vi "Initialize.vi"(7 "큐 입력":refnum<queue>, 8 "error in":errorcluster caption="에러 입력(에러 없음)", 11 "입력 클러스터":T1) -> (0 "error out":errorcluster caption="에러 출력", 2 "data 2 (3d)":string[][][](array[string]), 3 "data 1 (2d)":string[][](array[string]), 4 "Load?":bool)   [LabVIEW 2020]
uses:
  Controls/Clst_Initialize Input.ctl
  Controls/Cmd_Var Data IO.ctl
  Controls/Cmd_File path.ctl
  Controls/Cmd_File Type.ctl
  Variables/Global_Cal Info.vi
  Public/Polymorph/Table Initialize_2D.vi
  Public/Polymorph/Cell Space_Table.vi
  Public/Polymorph/String content_Str.vi
  Public/Polymorph/String content_Combo.vi
  Public/Polymorph/Table Initialize_Str.vi
  Public/Polymorph/Array Dedup_1D Str.vi
  Variables/Global_Cal STD.vi
  Public/Polymorph/Data Class_2D Str.vi
  <vilib>/Utility/file.llb/Read Delimited Spreadsheet (string).vi
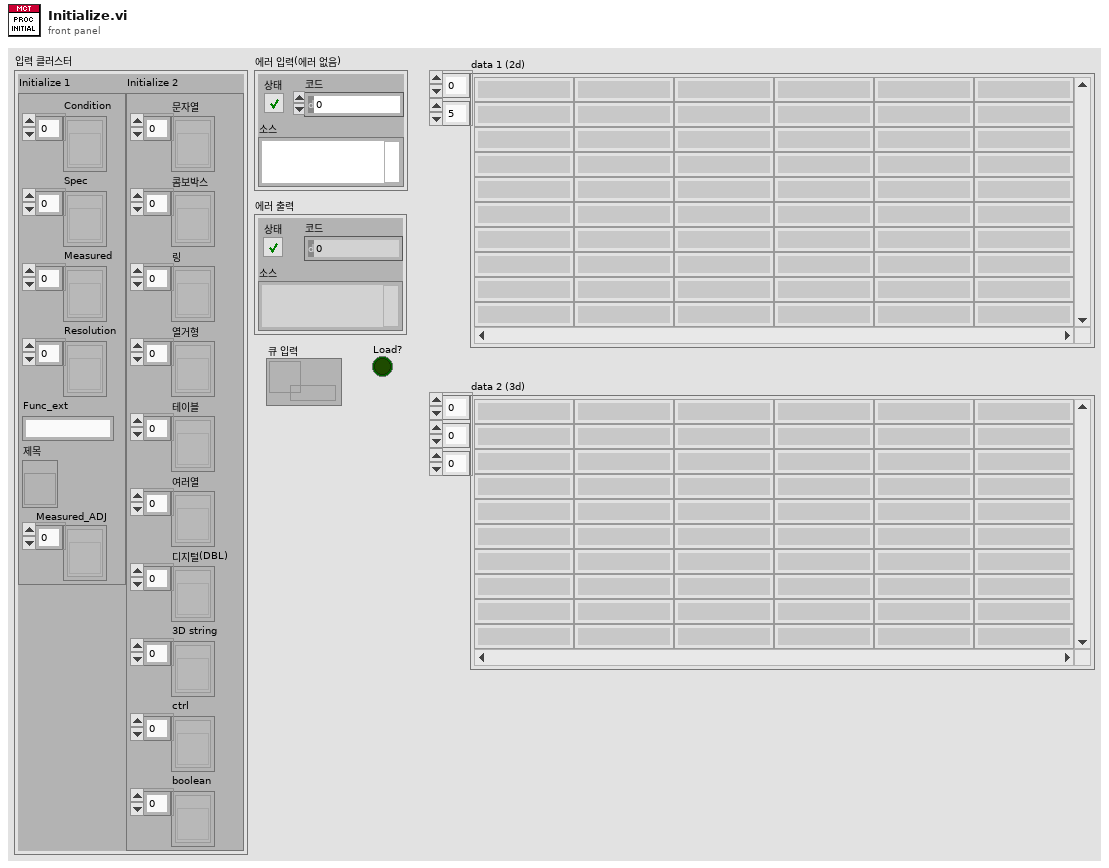
[diagram p1: front panel]
types:
  T1 = typedef "Clst_Initialize Input.ctl" = cluster{"Initialize 1":cluster{"Condition":refnum<vi>[], "Spec":refnum<vi>[], "Measured":refnum<vi>[], "Resolution":refnum<vi>[], "Func_ext":string, "제목":refnum<vi>, "Measured_ADJ":refnum<vi>[]}, "Initialize 2":cluster{"문자열":refnum<vi>[], "콤보박스":refnum<vi>[], "링":refnum<vi>[], "열거형":refnum<vi>[], "테이블":refnum<vi>[], "여러열":refnum<vi>[], "디지털(DBL)":refnum<vi>[], "3D string":refnum<vi>[], "ctrl":refnum<vi>[], "boolean":refnum<vi>[]}}
  T2 = cluster{"세부분류코드":string, "형식":string, "옵션":string, "측정기명":string, "EXCEL파일명":string, "TEMP":string}
  T3 = cluster{"Display sys":string[], "변경항목비활성":i32[], "추가항목비활성":i32[]}
  T4 = typedef "Cmd_Var Data IO.ctl" = enum16{"Condition", "Condition Default", "Condition_Temp", "Resolution", "Resolution Default", "Resolution Old", "Spec", "Spec Default", "Spec Old", "Spec Temp", "Result", "Result2", "Result3", "Result_Temp", "Result_ADJ", "Result_ADJ2", "STD1", "STD2", "STD3", "STD4", "STD5", "STD Temp", "CMC", "CMC Default"}
  T5 = enum8{"Enabled", "Disabled", "Disabled and Grayed Out"}
  T6 = typedef "Cmd_File Type.ctl" = enum16{"엑셀", "엑셀(2003)", "텍스트", "설정", "2진", "VI", "CSV", "LOG", "폴더"}
  T7 = typedef "Clst_Get Calproc.ctl" = cluster{"제목":string, "Condition":string[][], "Resolution":string[][], "Spec":string[][], "Data":string[][], "CMC":string[][], "NumRows":u32, "Temp_1":string[][]}
  T8 = typedef "Cmd_File path.ctl" = enum16{"에러로그", "데이터파일경로", "성적서원본", "지난성적서", "Data Files", "경로생성", "Updater", "Template", "설정파일경로", "FTP Upload", "Update 경로", "어플리케이션"}
  T9 = typedef "Clst_Cal Info Global.ctl" = cluster{"등록번호":string, "의뢰기관":string, "기기명":string, "제작회사":string, "형식":string, "기기번호":string, "소분류코드":string, "세부분류코드":string, "교정주기":string, "접수번호":string, "교정일자":string, "교정절차서 1":string, "교정절차서 2":string, "교정절차서 3":string, "접수확인자":string, "인증교정자":string, "기술책임자":string, "KOLAS 유무":string, "진행상태":string, "의뢰기관코드":string, "입고형태":string, "영문성적서?":bool, "합불판정?":bool, "부록?":bool, "절차서번호 1":string, "절차서번호 2":string, "절차서번호 3":string, "교정방식":string, "부서명":string}
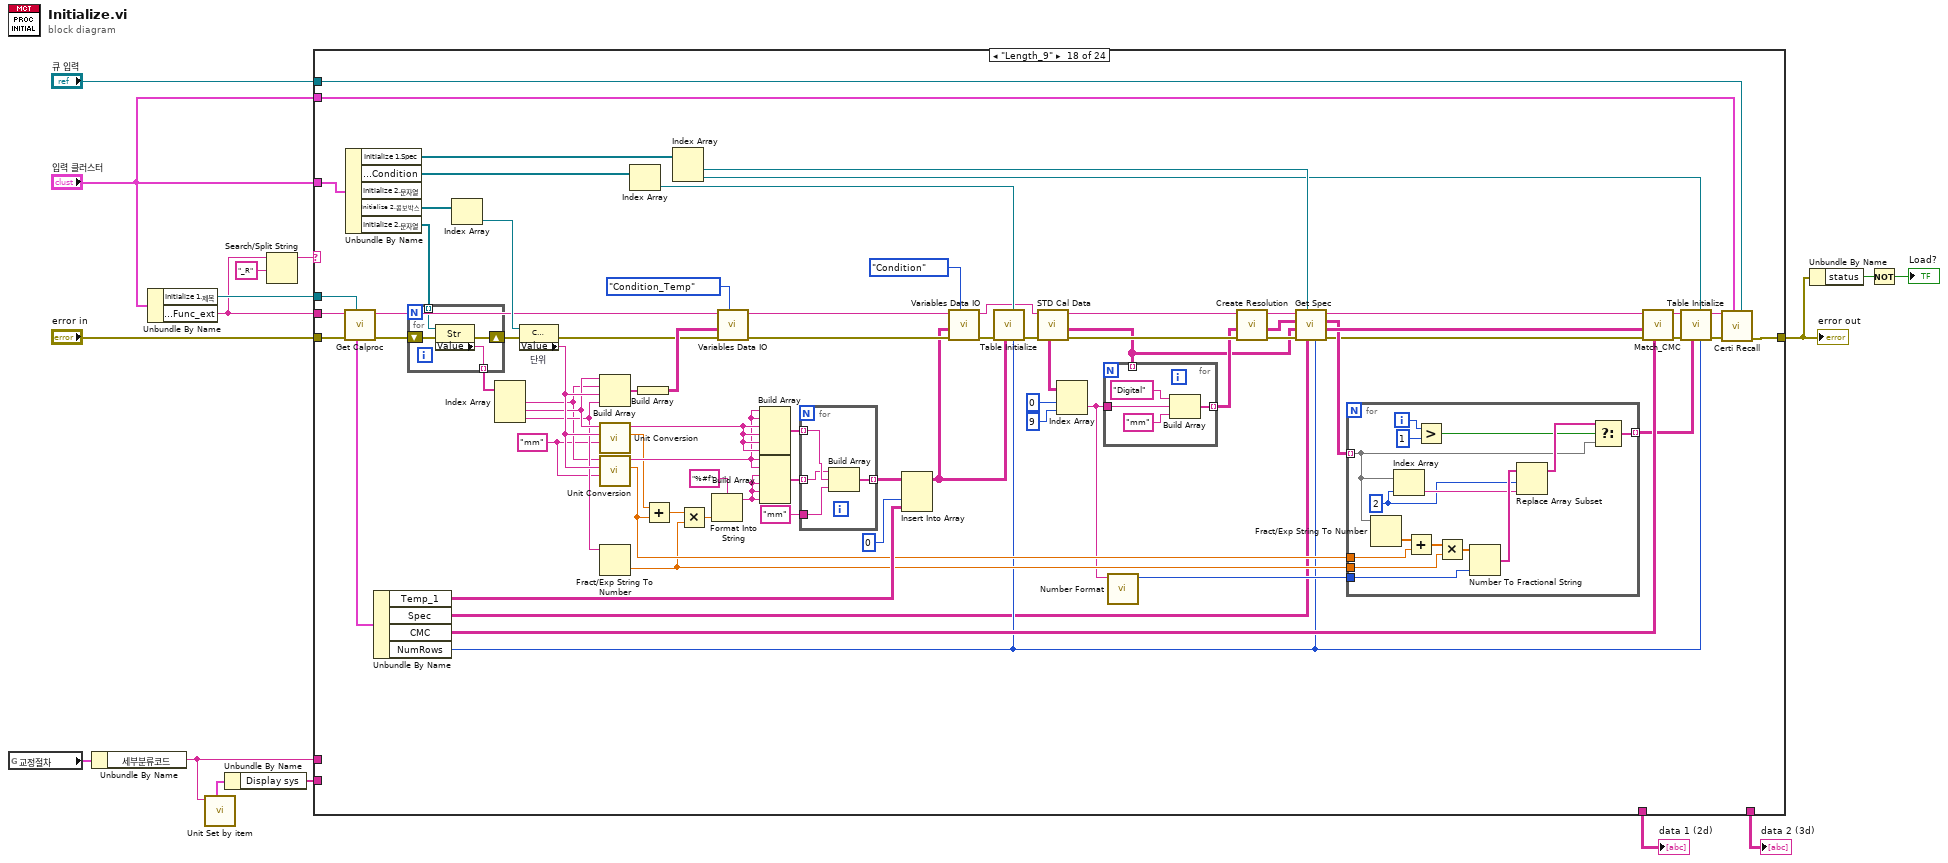
[diagram p0: block diagram]
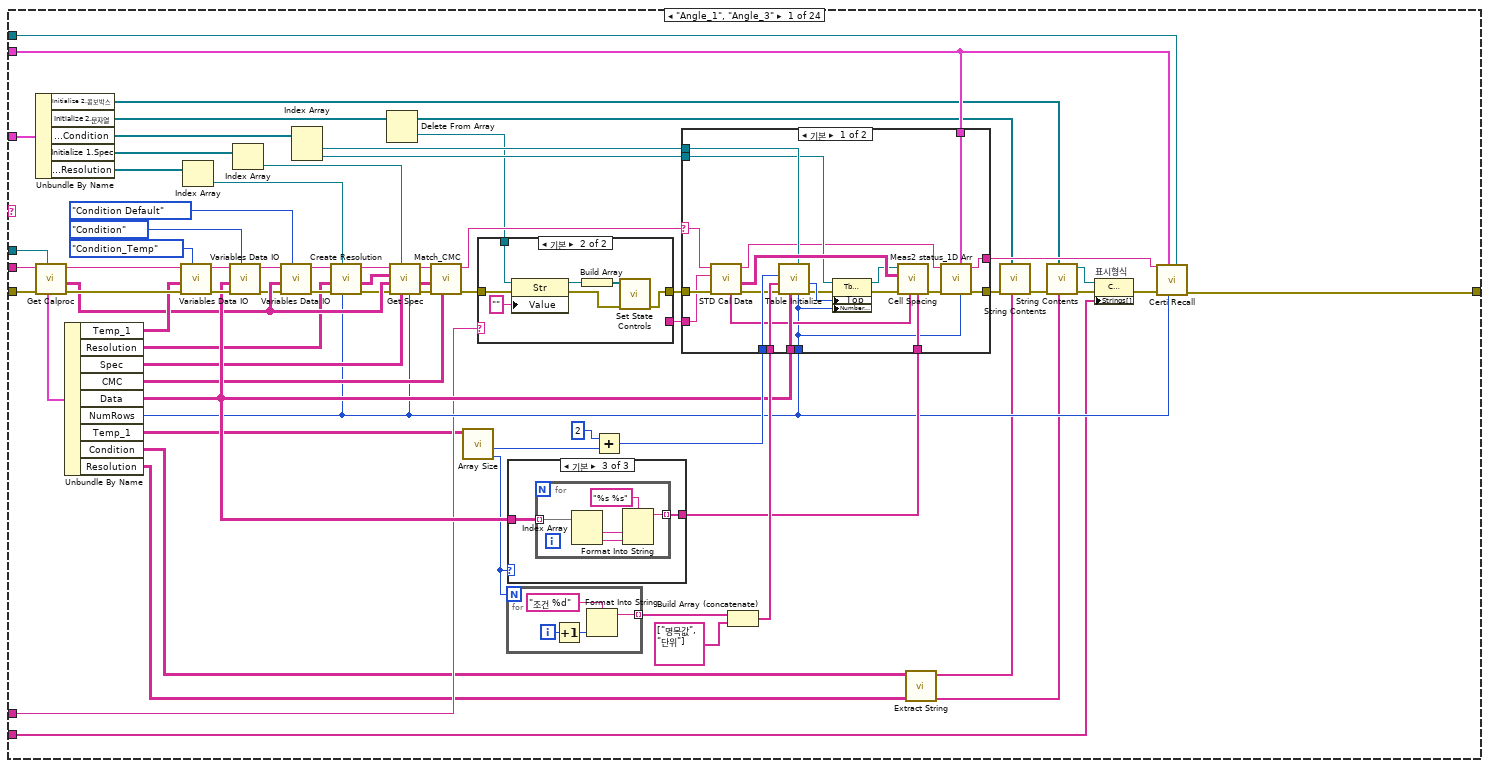
[diagram p2: hidden frame]
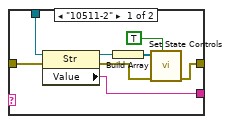
[diagram p3: hidden frame]
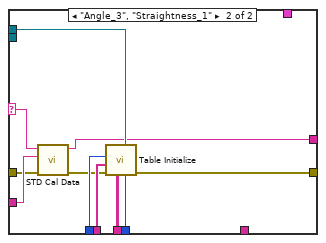
[diagram p4: hidden frame]
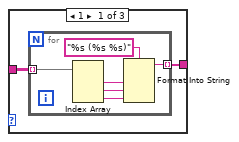
[diagram p5: hidden frame]
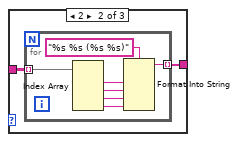
[diagram p6: hidden frame]
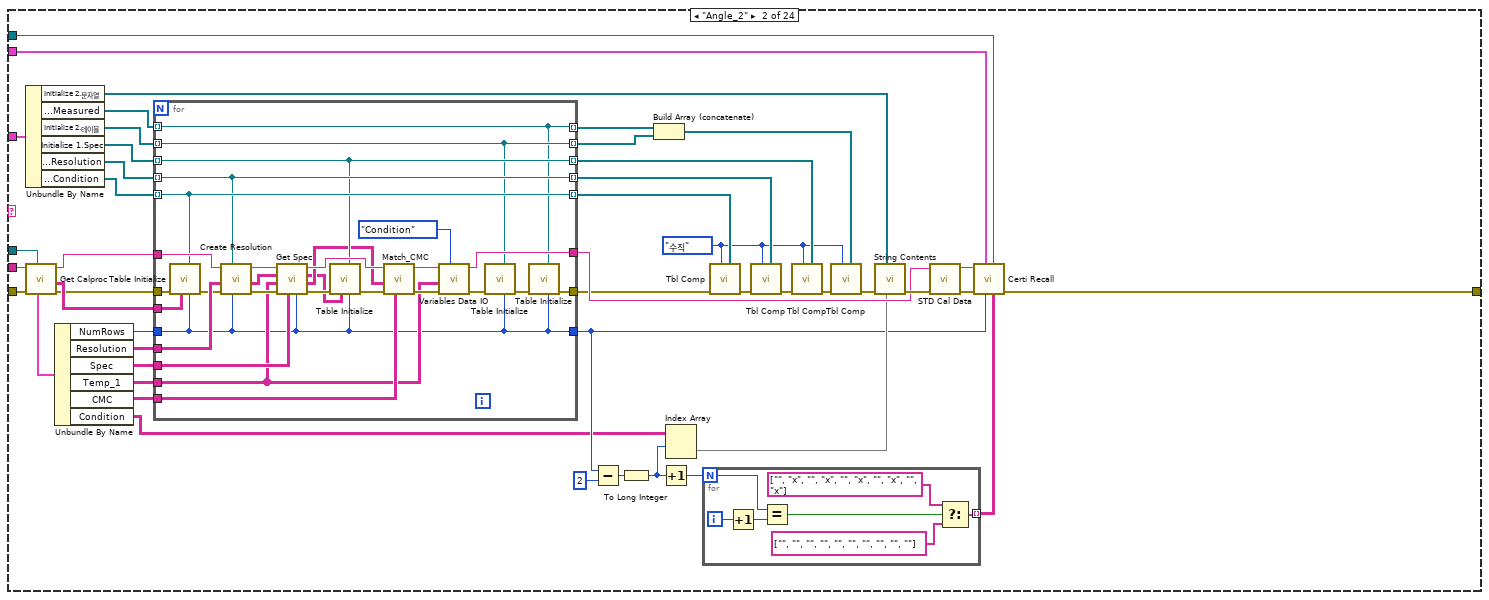
[diagram p7: hidden frame]
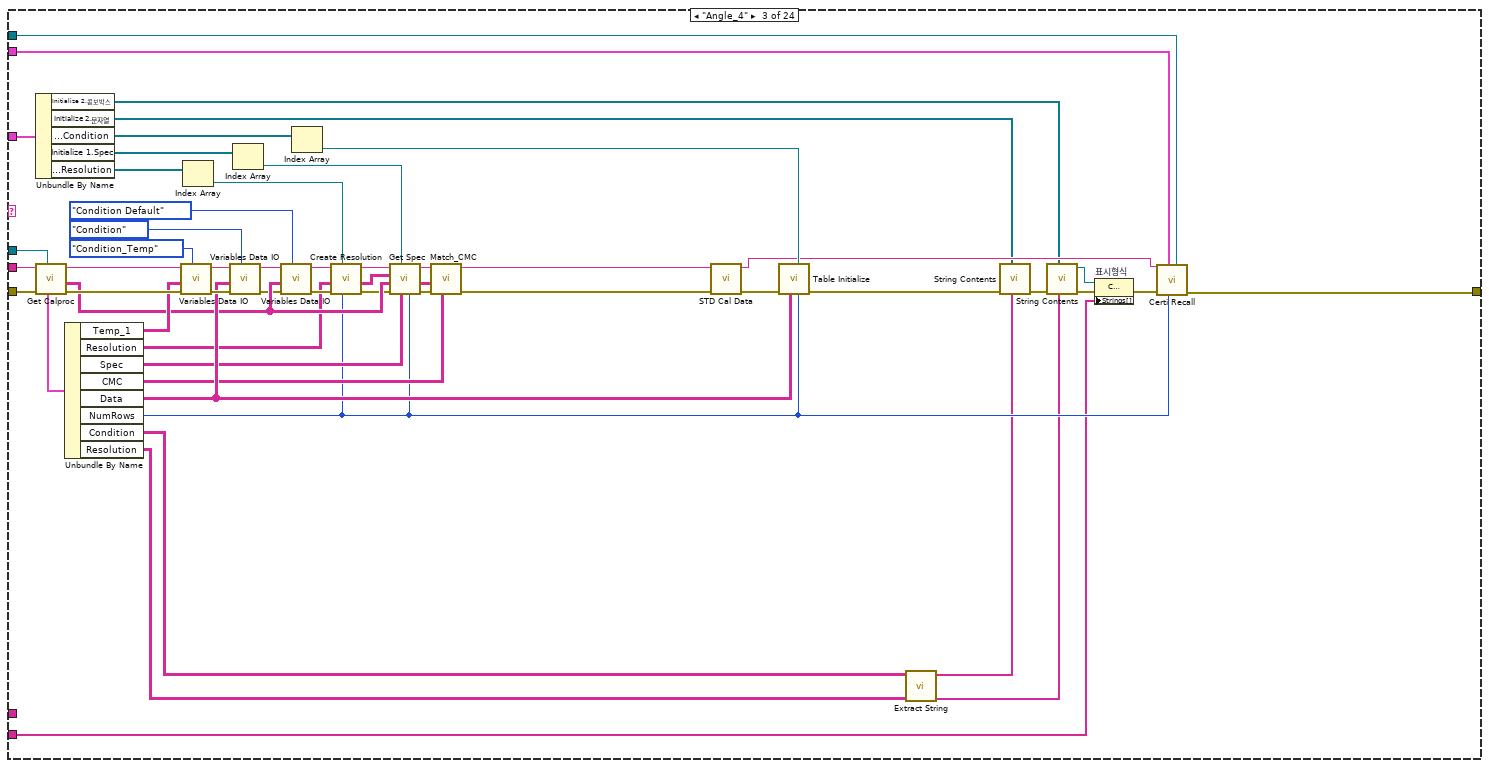
[diagram p8: hidden frame]
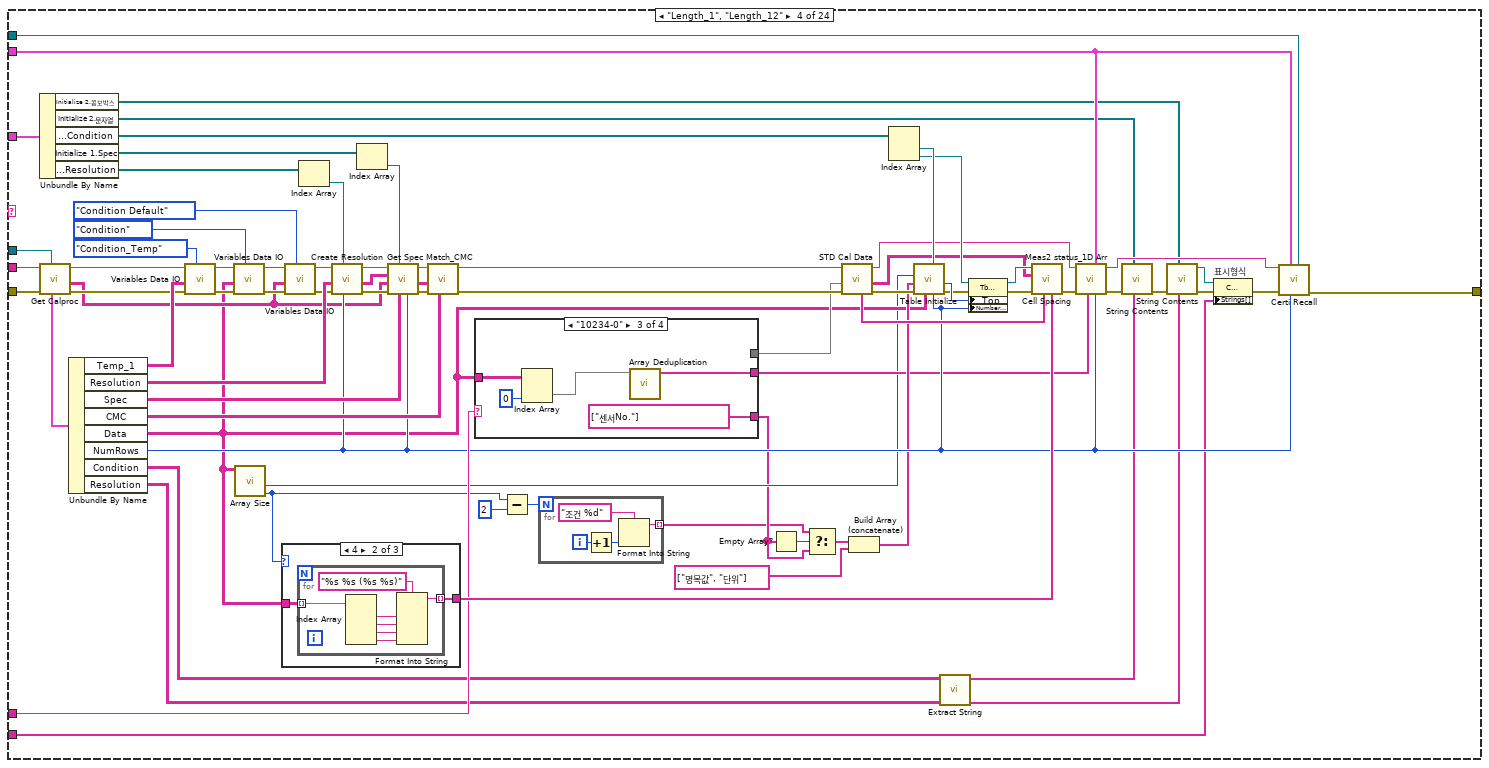
[diagram p9: hidden frame]
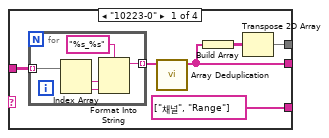
[diagram p10: hidden frame]
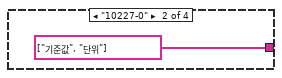
[diagram p11: hidden frame]
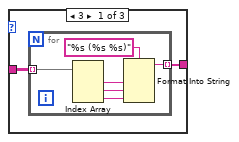
[diagram p13: hidden frame]
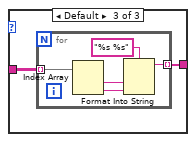
[diagram p14: hidden frame]
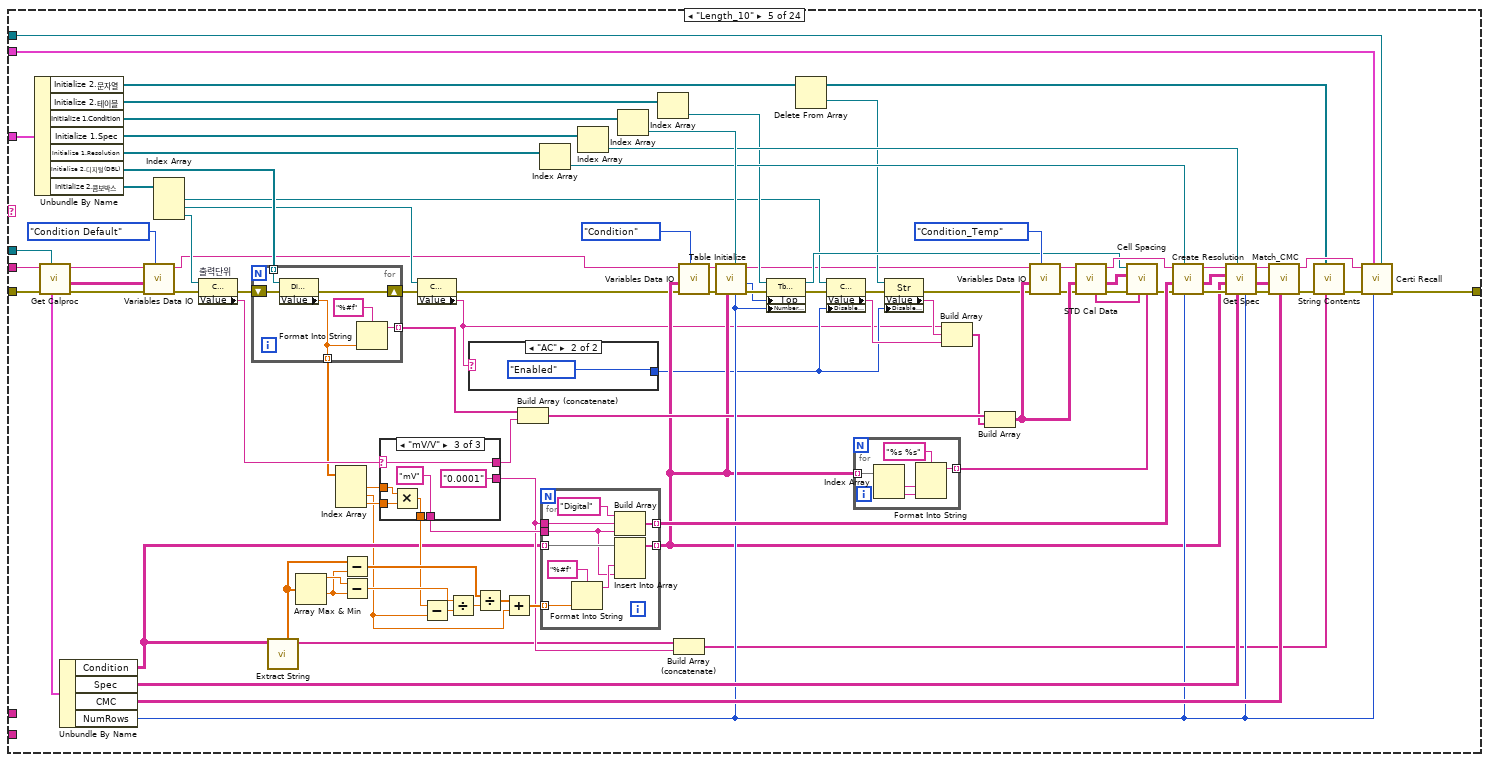
[diagram p15: hidden frame]
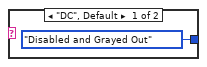
[diagram p16: hidden frame]
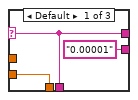
[diagram p17: hidden frame]
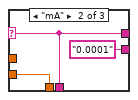
[diagram p18: hidden frame]
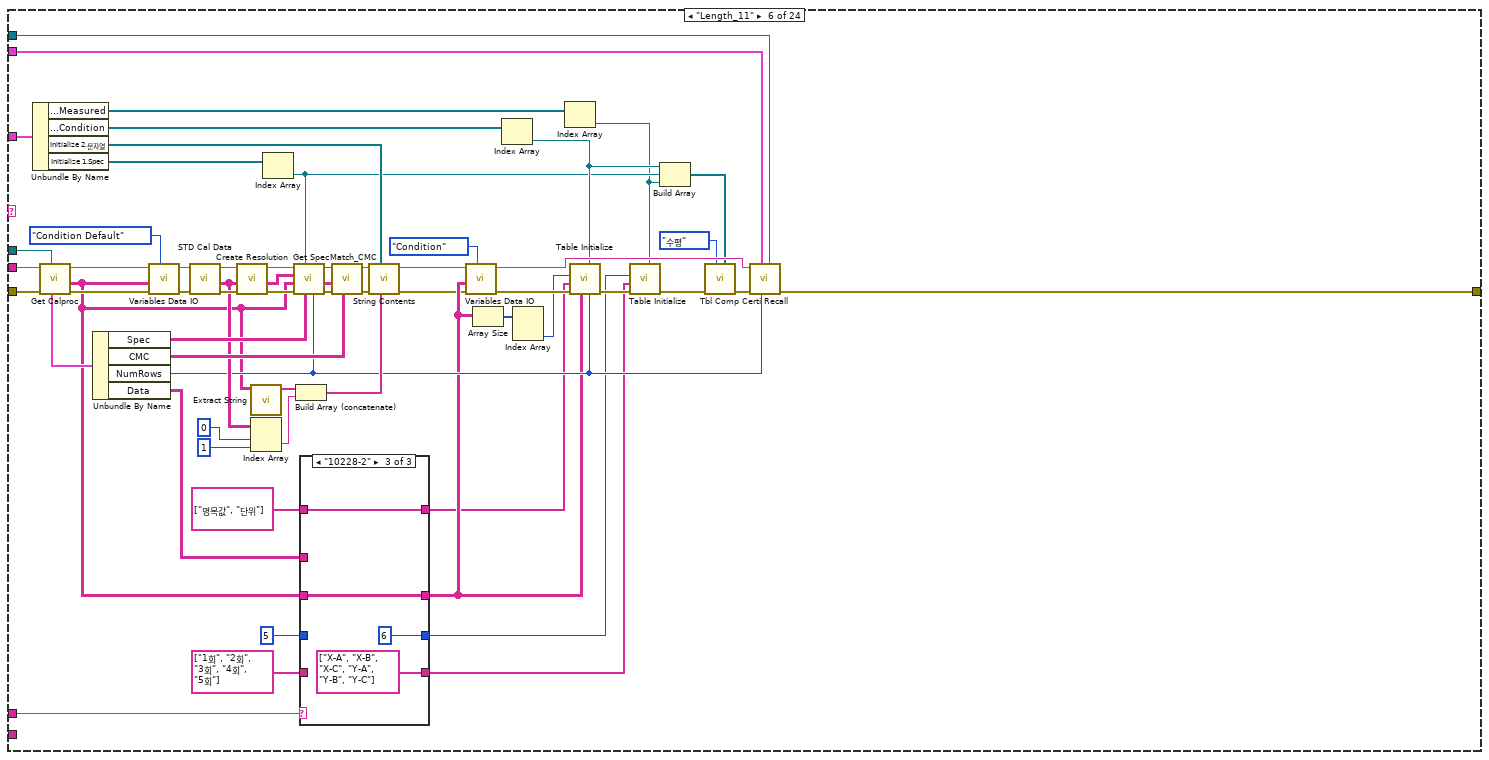
[diagram p19: hidden frame]
diagram:
  n1 = global read "Global_Cal Info.vi" "교정절차"() -> (w11:T2)
  n2 = Unbundle By Name(w11) -> ("세부분류코드"=w9:string)
  n3 = Unbundle By Name("입력 클러스터") -> ("Initialize 1.제목"=w10:refnum<vi>, "Initialize 1.Func_ext"=w2:string)
  n4 = call "Unit Set by item.vi"("분류코드"=w9) -> ("클러스터"=w8:T3)  [unwired: 3 in, 7 out]
  n5 = Unbundle By Name(w8) -> ("Display sys"=w7:string[])
  n6 = Search/Split String(string=w2, search string/char (-)="_R" ("검색 문자열/문자 (-)")) -> (substring before match=w12:string)  [unwired: 1 in, 2 out]
  n7 = case shown="\"Length_9\"" w12 {
    tunnel: "error in" -> [w45 w180 w263 w373 w511 w606 w694 w798 w881 w937 w1030 w1109 w1168 w1239 w1315 w1394 w1489 w1567 w1649 w1686 w1756 w1820 w1881 w1907]
    tunnel: [w44 w176 w262 w349 w487 w590 w681 w794 w847 w924 w1012 w1080 w1113 w1225 w1259 w1384 w1471 w1552 w1636 w1685 w1755 w1819 w1880 w1907] -> w6
    tunnel: "입력 클러스터" -> [w48 w179 w266 w360 w512 w600 w689 w773 w879 w931 w1022 w1086 w1161 w1229 w1306 w1386 w1476 w1564 w1641 w1689 w1759 w1823 w1884 _]
    tunnel: [_ _ _ _ _ _ _ w790 _ _ _ _ _ _ _ _ _ _ _ _ _ _ _ _] -> w16
    tunnel: "큐 입력" -> [w49 w178 w267 w348 w486 w594 w685 w795 w852 w926 w1011 w1079 w1147 w1224 w1304 w1383 w1470 w1554 w1635 w1690 w1760 w1824 w1885 _]
    tunnel: w2 -> [w46 w174 w264 w365 w510 w602 w691 w797 w880 w933 w1026 w1102 w1164 w1233 w1298 w1381 w1480 w1565 w1645 w1687 w1757 w1821 w1882 _]
    tunnel: w9 -> [w32 _ _ w336 _ w578 _ _ _ _ _ _ _ w1187 w1275 w1346 _ _ _ _ _ _ _ _]
    tunnel: "입력 클러스터" -> [w41 w177 w260 w321 w485 w595 w686 w796 w851 w927 w1005 w1052 w1148 w1190 w1303 w1350 w1446 w1553 w1634 w1683 w1753 w1817 w1878 _]
    tunnel: w10 -> [w47 w175 w265 w337 w509 w592 w683 w781 w877 w925 w1006 w1072 w1139 w1214 w1276 w1378 w1451 w1506 w1625 w1688 w1758 w1822 w1883 _]
    tunnel: w7 -> [w30 _ w254 w318 _ _ _ _ _ _ _ _ _ w1210 _ _ w1437 _ _ w1677 _ _ w1873 _]
    tunnel: [_ _ _ _ _ _ _ w786 _ _ _ _ _ _ _ _ _ _ _ _ _ _ _ _] -> w1
    frame "Angle_1", "Angle_3" {
      n8 = Unbundle By Name(w48) -> ("Initialize 2.콤보박스"=w17:refnum<vi>[], "Initialize 2.문자열"=w38:refnum<vi>[], "Initialize 1.Condition"=w39:refnum<vi>[], "Initialize 1.Spec"=w58:refnum<vi>[], "Initialize 1.Resolution"=w57:refnum<vi>[])
      n9 = call "Get Calproc.vi"("제목"=w47, "에러 입력"=w45, "Func_ext"=w46) -> ("에러 출력"=w79:errorcluster, "Condition"=w74:string[][], "Func_ext Out"=w77:string, "클러스터"=w69:T7)  [unwired: 5 in]
      n10 = Unbundle By Name(w69) -> ("Temp_1"=w76:string[][], "Resolution"=w66:string[][], "Spec"=w70:string[][], "CMC"=w59:string[][], "Data"=w75:string[][], "NumRows"=w42:u32, "Temp_1"=w31:string[][], "Condition"=w24:string[][], "Resolution"=w22:string[][])
      n11 = call "Variables Data IO.vi"("Select"=Cmd_Var_Data_IO."Condition_Temp", "error in"=w79, "Data In"=w76, "Func_ext"=w77) -> ("error out"=w80:errorcluster, "Func_ext Out"=w78:string)  [unwired: 5 in, 1 out]
      n12 = Index Array(array=w57) -> (element=w73:refnum<vi>)  [unwired: 1 in]
      n13 = call "Variables Data IO.vi"("Select"=Cmd_Var_Data_IO."Condition", "error in"=w80, "Data In"=w75, "Func_ext"=w78) -> ("error out"=w67:errorcluster, "Func_ext Out"=w54:string)  [unwired: 5 in, 1 out]
      n14 = Index Array(array=w58) -> (element=w63:refnum<vi>)  [unwired: 1 in]
      n15 = call "Variables Data IO.vi"("Select"=Cmd_Var_Data_IO."Condition Default", "error in"=w67, "Data In"=w74, "Func_ext"=w54) -> ("error out"=w81:errorcluster, "Func_ext Out"=w82:string)  [unwired: 5 in, 1 out]
      n16 = Index Array(array=w39) -> (element #1=w61:refnum<vi>, element #2=w43:refnum<vi>)  [unwired: 2 in]
      n17 = call "Create Resolution.vi"("행의 개수"=w42, "Table Ref"=w73, "에러 입력(에러 없음)"=w81, "Resolution"=w66, "Func_ext"=w82) -> ("에러 출력"=w53:errorcluster, "Resolution Out"=w71:string[][], "Func_ext 출력"=w72:string)  [unwired: 4 in]
      n18 = Delete From Array(array=w38) -> (deleted portion=w35:refnum<vi>, array with subset deleted=w27:refnum<vi>[])  [unwired: 2 in]
      n19 = call "Get Spec.vi"("NumRows"=w42, "Spec in"=w70, "Spec Ref."=w63, "error in"=w53, "Condition in"=w74, "Resolution in"=w71, "Func_ext"=w72) -> ("error out"=w52:errorcluster, "Data Out"=w56:string[][], "Func_ext Out"=w55:string)  [unwired: 2 out]
      n20 = call "Match_CMC.vi"("CMC IN"=w59, "error in"=w52, "Condition IN"=w56, "Func_ext"=w55) -> ("error out"=w37:errorcluster, "Func_ext out"=w36:string)  [unwired: 4 in, 2 out]
      n21 = call "Array Size.vi"("Data in"=w31) -> ("열(I32)"=w26:i32, "열(U32)"=w18:u32)  [unwired: 7 in, 2 out]
      n22 = case shown="기본" w32 {
        tunnel: w37 -> [w90 w98]
        tunnel: w35 -> [w89 w97]
        tunnel: [w92 _] -> w34
        tunnel: [w86 w94] -> w33
        frame "10511-2" {
          n23 = property class="Str"(reference=w89, error in=w90) -> (reference out=w88:refnum<vi>, error out=w87:errorcluster, "Value"=w92:string)
          n24 = Build Array(w88) -> (w91:refnum<vi>[])
          n25 = call "Set State Controls.vi"("활성화 (F)"=TRUE, "error in (no error)"=w87, "컨트롤 참조 배열 in"=w91) -> ("error out"=w86:errorcluster)  [unwired: 7 in, 1 out]
        }
        frame Default {
          n26 = property class="Str"(reference=w97, error in=w98, "Value"="" ("값")) -> (reference out=w96:refnum<vi>, error out=w95:errorcluster)
          n27 = Build Array(w96) -> (w99:refnum<vi>[])
          n28 = call "Set State Controls.vi"("error in (no error)"=w95, "컨트롤 참조 배열 in"=w99) -> ("error out"=w94:errorcluster)  [unwired: 8 in, 1 out]
        }
      }
      n29 = for {
        N: w26 -> [_]
        tunnel: [w133] -> w64 mode=indexing
        i -> [w136]
        n30 = Increment(x=w136) -> (x+1=w135:i32)
        n31 = Format Into String(format string="조건 %d" ("포맷 문자열"), w135) -> (resulting string=w133:string)  [unwired: 2 in, 1 out]
      }
      n32 = case shown="기본" w26 {
        tunnel: w75 -> [w138 w146 w155]
        tunnel: [w137 w145 w154] -> w60
        frame 1 {
          n33 = for {
            tunnel: w138 -> [w144] mode=indexing
            tunnel: [w139] -> w137 mode=indexing
            n34 = Index Array(array=w144) -> (element #1=w143:string, element #2=w142:string, element #3=w141:string)  [unwired: 3 in]
            n35 = Format Into String(format string="%s (%s %s)" ("포맷 문자열"), w143, w142, w141) -> (resulting string=w139:string)  [unwired: 2 in, 1 out]
          }
        }
        frame 2 {
          n36 = for {
            tunnel: w146 -> [w153] mode=indexing
            tunnel: [w148] -> w145 mode=indexing
            n37 = Index Array(array=w153) -> (element #1=w152:string, element #2=w151:string, element #3=w150:string, element #4=w147:string)  [unwired: 4 in]
            n38 = Format Into String(format string="%s %s (%s %s)" ("포맷 문자열"), w152, w151, w150, w147) -> (resulting string=w148:string)  [unwired: 2 in, 1 out]
          }
        }
        frame Default {
          n39 = for {
            tunnel: w155 -> [w160] mode=indexing
            tunnel: [w156] -> w154 mode=indexing
            n40 = Index Array(array=w160) -> (element #1=w159:string, element #2=w158:string)  [unwired: 2 in]
            n41 = Format Into String(format string="%s %s" ("포맷 문자열"), w159, w158) -> (resulting string=w156:string)  [unwired: 2 in, 1 out]
          }
        }
      }
      n42 = Add(x=u32 2 ("y"), y=w18) -> (x+y=w83:u32)
      n43 = Build Array (concatenate)(w64, string[] ["명목값", "단위"]) -> (w84:string[])
      n44 = case shown="기본" w36 {
        selector: w36 -> [w102 w124]
        tunnel: w84 -> [w121 w132]
        tunnel: w83 -> [w120 w131]
        tunnel: w75 -> [w119 w130]
        tunnel: w61 -> [w115 w128]
        tunnel: w60 -> [w114 _]
        tunnel: w43 -> [w111 _]
        tunnel: w42 -> [w109 w126]
        tunnel: w41 -> [w108 _]
        tunnel: [w107 w125] -> w21
        tunnel: [w106 w127] -> w40
        tunnel: w33 -> [w105 w122]
        tunnel: w34 -> [w101 w123]
        frame Default {
          n45 = call "STD Cal Data.vi"("error in"=w105, "문자열"=w101, "Func_ext"=w102) -> ("error out"=w116:errorcluster, "Data Out"=w118:string[][], "Func_ext Out"=w110:string, "Data Out 2"=w117:string[])  [unwired: 4 in, 1 out]
          n46 = call-poly "Table Initialize.vi"("행의 개수"=w109, "Table Ref"=w115, "Value"=w119, "에러 입력"=w116, "열해더 문자열"=w121, "열의 개수"=w120) -> ("에러 출력"=w112:errorcluster, "Bottom"=w113:i32)  [unwired: 3 in, 1 out]
          n47 = property class="Tbl (엄격한)"(reference=w111, error in=w112, "Top"=w113, "Number of Rows"=w109) -> (reference out=w100:refnum<vi>, error out=w104:errorcluster)
          n48 = call-poly "Cell Spacing.vi"("Row Header in"=w114, "Col Header in"=w117, "error in"=w104, "Data in"=w118, "테이블 참조 in"=w100) -> ("error out"=w103:errorcluster)  [unwired: 4 in, 2 out]
          n49 = call "Meas2 status_1D Arr.vi"("행의 개수"=w109, "입력 클러스터"=w108, "에러 입력"=w103, "Func_ext"=w110) -> ("에러 출력"=w107:errorcluster, "Func_ext Out"=w106:string)  [unwired: 6 in]
        }
        frame "Angle_3", "Straightness_1" {
          n50 = call "STD Cal Data.vi"("error in"=w122, "문자열"=w123, "Func_ext"=w124) -> ("error out"=w129:errorcluster, "Func_ext Out"=w127:string)  [unwired: 4 in, 3 out]
          n51 = call-poly "Table Initialize.vi"("행의 개수"=w126, "Table Ref"=w128, "Value"=w130, "에러 입력"=w129, "열해더 문자열"=w132, "열의 개수"=w131) -> ("에러 출력"=w125:errorcluster)  [unwired: 3 in, 2 out]
        }
      }
      n52 = call "Extract String.vi"("Resolution"=w22, "Condition"=w24) -> ("배열 1"=w25:string[], "배열 2"=w23:string[])  [unwired: 7 in, 1 out]
      n53 = call-poly "String Contents.vi"("문자 배열"=w23, "참조 배열"=w27, "에러 입력"=w21) -> ("에러 출력"=w20:errorcluster)  [unwired: 7 in, 1 out]
      n54 = call-poly "String Contents.vi"("문자 배열"=w25, "참조 배열"=w17, "에러 입력"=w20) -> ("에러 출력"=w29:errorcluster, "참조"=w28:refnum<vi>)  [unwired: 7 in]
      n55 = property on="표시형식" class="CmbBox"(reference=w28, error in=w29, "Strings[]"=w30) -> (error out=w19:errorcluster)  [unwired: 1 out]
      n56 = call "Certi Recall.vi"("큐 입력"=w49, "NumRows"=w42, "입력 클러스터"=w41, "에러 입력"=w19, "Func_ext in"=w40) -> ("에러 출력"=w44:errorcluster)  [unwired: 5 in, 1 out]
    }
    frame "Angle_2" {
      w166 = enum16{"수직", "수평"}."수직" ("방향")
      n57 = Unbundle By Name(w179) -> ("Initialize 2.문자열"=w165:refnum<vi>[], "Initialize 1.Measured"=w162:refnum<vi>[], "Initialize 2.테이블"=w164:refnum<vi>[], "Initialize 1.Spec"=w188:refnum<vi>[], "Initialize 1.Resolution"=w185:refnum<vi>[], "Initialize 1.Condition"=w183:refnum<vi>[])
      n58 = call "Get Calproc.vi"("제목"=w175, "에러 입력"=w180, "Func_ext"=w174) -> ("에러 출력"=w181:errorcluster, "Condition"=w206:string[][], "Func_ext Out"=w187:string, "클러스터"=w182:T7)  [unwired: 5 in]
      n59 = Unbundle By Name(w182) -> ("NumRows"=w184:u32, "Resolution"=w186:string[][], "Spec"=w189:string[][], "Temp_1"=w190:string[][], "CMC"=w191:string[][], "Condition"=w173:string[][])
      n60 = for {
        tunnel: w183 -> [w232] mode=indexing
        tunnel: w181 -> [w242]
        tunnel: w206 -> [w222]
        tunnel: w184 -> [w216]
        tunnel: w185 -> [w228] mode=indexing
        tunnel: w186 -> [w241]
        tunnel: w187 -> [w237]
        tunnel: w188 -> [w226] mode=indexing
        tunnel: w189 -> [w231]
        tunnel: w190 -> [w221]
        tunnel: w191 -> [w239]
        tunnel: [w216] -> w192
        tunnel: [w217] -> w195
        tunnel: [w233] -> w202
        tunnel: [w232] -> w172 mode=indexing
        tunnel: [w228] -> w171 mode=indexing
        tunnel: [w226] -> w170 mode=indexing
        tunnel: w164 -> [w219] mode=indexing
        tunnel: [w219] -> w163 mode=indexing
        tunnel: w162 -> [w215] mode=indexing
        tunnel: [w215] -> w161 mode=indexing
        n61 = call-poly "Table Initialize.vi"("행의 개수"=w216, "Table Ref"=w232, "Value"=w222, "에러 입력"=w242) -> ("에러 출력"=w238:errorcluster)  [unwired: 5 in, 2 out]
        n62 = call "Create Resolution.vi"("행의 개수"=w216, "Table Ref"=w228, "에러 입력(에러 없음)"=w238, "Resolution"=w241, "Func_ext"=w237) -> ("에러 출력"=w227:errorcluster, "Resolution Out"=w230:string[][], "Func_ext 출력"=w229:string)  [unwired: 4 in]
        n63 = call "Get Spec.vi"("NumRows"=w216, "Spec in"=w231, "error in"=w227, "Condition in"=w221, "Resolution in"=w230, "Func_ext"=w229) -> ("error out"=w225:errorcluster, "Data Out"=w223:string[][], "Spec Out"=w214:string[][], "Func_ext Out"=w240:string)  [unwired: 1 in, 1 out]
        n64 = call-poly "Table Initialize.vi"("행의 개수"=w216, "Table Ref"=w226, "Value"=w214, "에러 입력"=w225) -> ("에러 출력"=w224:errorcluster)  [unwired: 5 in, 2 out]
        n65 = call "Match_CMC.vi"("CMC IN"=w239, "error in"=w224, "Condition IN"=w223, "Func_ext"=w240) -> ("error out"=w235:errorcluster, "Func_ext out"=w236:string)  [unwired: 4 in, 2 out]
        n66 = call "Variables Data IO.vi"("Select"=Cmd_Var_Data_IO."Condition", "error in"=w235, "Data In"=w221, "Func_ext"=w236) -> ("error out"=w220:errorcluster, "Func_ext Out"=w233:string)  [unwired: 5 in, 1 out]
        n67 = call-poly "Table Initialize.vi"("행의 개수"=w216, "Table Ref"=w219, "에러 입력"=w220) -> ("에러 출력"=w218:errorcluster)  [unwired: 6 in, 2 out]
        n68 = call-poly "Table Initialize.vi"("행의 개수"=w216, "Table Ref"=w215, "에러 입력"=w218) -> ("에러 출력"=w217:errorcluster)  [unwired: 6 in, 2 out]
      }
      n69 = Subtract(x=w192, y=u32 2) -> (x-y=w198:u32)
      n70 = To Long Integer(number=w198) -> (32bit integer=w199:i32)
      n71 = Build Array (concatenate)(w161, w163) -> (w167:refnum<vi>[])
      n72 = Increment(x=w199) -> (x+1=w201:i32)
      n73 = Index Array(array=w173, index (row)=w199) -> (element=w194:string[])  [unwired: 1 in]
      n74 = for {
        N: w201 -> [w213]
        tunnel: [w207] -> w200 mode=indexing
        i -> [w212]
        n75 = Increment(x=w212) -> (x+1=w211:i32)
        n76 = Equal?(x=w213, y=w211) -> (x = y?=w210:bool)
        n77 = Select(t=string[] ["", "ⅹ", "", "ⅹ", "", "ⅹ", "", "ⅹ", "", "ⅹ"], s=w210, f=string[] ["", "", "", "", "", "", "", "", "", ""]) -> (s? t:f=w207:string[])
      }
      n78 = call "Tbl Comp.vi"("배열"=w172, "방향"=w166, "에러 입력"=w195) -> ("에러 출력"=w196:errorcluster)  [unwired: 6 in, 2 out]
      n79 = call "Tbl Comp.vi"("배열"=w171, "방향"=w166, "에러 입력"=w196) -> ("에러 출력"=w197:errorcluster)  [unwired: 6 in, 2 out]
      n80 = call "Tbl Comp.vi"("배열"=w170, "방향"=w166, "에러 입력"=w197) -> ("에러 출력"=w169:errorcluster)  [unwired: 6 in, 2 out]
      n81 = call "Tbl Comp.vi"("배열"=w167, "방향"=w166, "에러 입력"=w169) -> ("에러 출력"=w168:errorcluster)  [unwired: 6 in, 2 out]
      n82 = call-poly "String Contents.vi"("문자 배열"=w194, "참조 배열"=w165, "에러 입력"=w168) -> ("에러 출력"=w205:errorcluster)  [unwired: 7 in, 1 out]
      n83 = call "STD Cal Data.vi"("error in"=w205, "Func_ext"=w202) -> ("error out"=w204:errorcluster, "Func_ext Out"=w203:string)  [unwired: 5 in, 3 out]
      n84 = call "Certi Recall.vi"("Value"=w200, "큐 입력"=w178, "NumRows"=w192, "입력 클러스터"=w177, "에러 입력"=w204, "Func_ext in"=w203) -> ("에러 출력"=w176:errorcluster)  [unwired: 4 in, 1 out]
    }
    frame "Angle_4" {
      n85 = Unbundle By Name(w266) -> ("Initialize 2.콤보박스"=w244:refnum<vi>[], "Initialize 2.문자열"=w257:refnum<vi>[], "Initialize 1.Condition"=w258:refnum<vi>[], "Initialize 1.Spec"=w276:refnum<vi>[], "Initialize 1.Resolution"=w275:refnum<vi>[])
      n86 = call "Get Calproc.vi"("제목"=w265, "에러 입력"=w263, "Func_ext"=w264) -> ("에러 출력"=w293:errorcluster, "Condition"=w288:string[][], "Func_ext Out"=w291:string, "클러스터"=w283:T7)  [unwired: 5 in]
      n87 = Unbundle By Name(w283) -> ("Temp_1"=w290:string[][], "Resolution"=w280:string[][], "Spec"=w284:string[][], "CMC"=w277:string[][], "Data"=w289:string[][], "NumRows"=w261:u32, "Condition"=w250:string[][], "Resolution"=w248:string[][])
      n88 = call "Variables Data IO.vi"("Select"=Cmd_Var_Data_IO."Condition_Temp", "error in"=w293, "Data In"=w290, "Func_ext"=w291) -> ("error out"=w294:errorcluster, "Func_ext Out"=w292:string)  [unwired: 5 in, 1 out]
      n89 = Index Array(array=w275) -> (element=w287:refnum<vi>)  [unwired: 1 in]
      n90 = call "Variables Data IO.vi"("Select"=Cmd_Var_Data_IO."Condition", "error in"=w294, "Data In"=w289, "Func_ext"=w292) -> ("error out"=w281:errorcluster, "Func_ext Out"=w272:string)  [unwired: 5 in, 1 out]
      n91 = Index Array(array=w276) -> (element=w279:refnum<vi>)  [unwired: 1 in]
      n92 = call "Variables Data IO.vi"("Select"=Cmd_Var_Data_IO."Condition Default", "error in"=w281, "Data In"=w288, "Func_ext"=w272) -> ("error out"=w295:errorcluster, "Func_ext Out"=w296:string)  [unwired: 5 in, 1 out]
      n93 = Index Array(array=w258) -> (element=w278:refnum<vi>)  [unwired: 1 in]
      n94 = call "Create Resolution.vi"("행의 개수"=w261, "Table Ref"=w287, "에러 입력(에러 없음)"=w295, "Resolution"=w280, "Func_ext"=w296) -> ("에러 출력"=w271:errorcluster, "Resolution Out"=w285:string[][], "Func_ext 출력"=w286:string)  [unwired: 4 in]
      n95 = call "Get Spec.vi"("NumRows"=w261, "Spec in"=w284, "Spec Ref."=w279, "error in"=w271, "Condition in"=w288, "Resolution in"=w285, "Func_ext"=w286) -> ("error out"=w270:errorcluster, "Data Out"=w274:string[][], "Func_ext Out"=w273:string)  [unwired: 2 out]
      n96 = call "Match_CMC.vi"("CMC IN"=w277, "error in"=w270, "Condition IN"=w274, "Func_ext"=w273) -> ("error out"=w256:errorcluster, "Func_ext out"=w255:string)  [unwired: 4 in, 2 out]
      n97 = call "STD Cal Data.vi"("error in"=w256, "Func_ext"=w255) -> ("error out"=w243:errorcluster, "Func_ext Out"=w259:string)  [unwired: 5 in, 3 out]
      n98 = call-poly "Table Initialize.vi"("행의 개수"=w261, "Table Ref"=w278, "Value"=w289, "에러 입력"=w243) -> ("에러 출력"=w247:errorcluster)  [unwired: 5 in, 2 out]
      n99 = call "Extract String.vi"("Resolution"=w248, "Condition"=w250) -> ("배열 1"=w251:string[], "배열 2"=w249:string[])  [unwired: 7 in, 1 out]
      n100 = call-poly "String Contents.vi"("문자 배열"=w249, "참조 배열"=w257, "에러 입력"=w247) -> ("에러 출력"=w246:errorcluster)  [unwired: 7 in, 1 out]
      n101 = call-poly "String Contents.vi"("문자 배열"=w251, "참조 배열"=w244, "에러 입력"=w246) -> ("에러 출력"=w253:errorcluster, "참조"=w252:refnum<vi>)  [unwired: 7 in]
      n102 = property on="표시형식" class="CmbBox"(reference=w252, error in=w253, "Strings[]"=w254) -> (error out=w245:errorcluster)  [unwired: 1 out]
      n103 = call "Certi Recall.vi"("큐 입력"=w267, "NumRows"=w261, "입력 클러스터"=w260, "에러 입력"=w245, "Func_ext in"=w259) -> ("에러 출력"=w262:errorcluster)  [unwired: 5 in, 1 out]
    }
    frame "Length_1", "Length_12" {
      n104 = Unbundle By Name(w360) -> ("Initialize 2.콤보박스"=w316:refnum<vi>[], "Initialize 2.문자열"=w302:refnum<vi>[], "Initialize 1.Condition"=w307:refnum<vi>[], "Initialize 1.Spec"=w306:refnum<vi>[], "Initialize 1.Resolution"=w308:refnum<vi>[])
      n105 = call "Get Calproc.vi"("제목"=w337, "에러 입력"=w373, "Func_ext"=w365) -> ("에러 출력"=w332:errorcluster, "Condition"=w322:string[][], "Func_ext Out"=w334:string, "클러스터"=w350:T7)  [unwired: 5 in]
      n106 = Unbundle By Name(w350) -> ("Temp_1"=w335:string[][], "Resolution"=w356:string[][], "Spec"=w341:string[][], "CMC"=w363:string[][], "Data"=w314:string[][], "NumRows"=w328:u32, "Condition"=w310:string[][], "Resolution"=w301:string[][])
      n107 = call "Variables Data IO.vi"("Select"=Cmd_Var_Data_IO."Condition_Temp", "error in"=w332, "Data In"=w335, "Func_ext"=w334) -> ("error out"=w331:errorcluster, "Func_ext Out"=w333:string)  [unwired: 5 in, 1 out]
      n108 = call "Variables Data IO.vi"("Select"=Cmd_Var_Data_IO."Condition", "error in"=w331, "Data In"=w314, "Func_ext"=w333) -> ("error out"=w355:errorcluster, "Func_ext Out"=w368:string)  [unwired: 5 in, 1 out]
      n109 = call "Array Size.vi"("Data in"=w314) -> ("열(I32)"=w313:i32, "열(U32)"=w312:u32)  [unwired: 7 in, 2 out]
      n110 = case shown="4" w313 {
        tunnel: w314 -> [w396 w404 w413]
        tunnel: [w395 w403 w412] -> w361
        frame 3 {
          n111 = for {
            tunnel: w396 -> [w402] mode=indexing
            tunnel: [w397] -> w395 mode=indexing
            n112 = Index Array(array=w402) -> (element #1=w401:string, element #2=w400:string, element #3=w399:string)  [unwired: 3 in]
            n113 = Format Into String(format string="%s (%s %s)" ("포맷 문자열"), w401, w400, w399) -> (resulting string=w397:string)  [unwired: 2 in, 1 out]
          }
        }
        frame 4 {
          n114 = for {
            tunnel: w404 -> [w411] mode=indexing
            tunnel: [w406] -> w403 mode=indexing
            n115 = Index Array(array=w411) -> (element #1=w410:string, element #2=w409:string, element #3=w408:string, element #4=w405:string)  [unwired: 4 in]
            n116 = Format Into String(format string="%s %s (%s %s)" ("포맷 문자열"), w410, w409, w408, w405) -> (resulting string=w406:string)  [unwired: 2 in, 1 out]
          }
        }
        frame Default {
          n117 = for {
            tunnel: w413 -> [w418] mode=indexing
            tunnel: [w414] -> w412 mode=indexing
            n118 = Index Array(array=w418) -> (element #1=w417:string, element #2=w416:string)  [unwired: 2 in]
            n119 = Format Into String(format string="%s %s" ("포맷 문자열"), w417, w416) -> (resulting string=w414:string)  [unwired: 2 in, 1 out]
          }
        }
      }
      n120 = call "Variables Data IO.vi"("Select"=Cmd_Var_Data_IO."Condition Default", "error in"=w355, "Data In"=w322, "Func_ext"=w368) -> ("error out"=w330:errorcluster, "Func_ext Out"=w329:string)  [unwired: 5 in, 1 out]
      n121 = Index Array(array=w308) -> (element=w338:refnum<vi>)  [unwired: 1 in]
      n122 = call "Create Resolution.vi"("행의 개수"=w328, "Table Ref"=w338, "에러 입력(에러 없음)"=w330, "Resolution"=w356, "Func_ext"=w329) -> ("에러 출력"=w369:errorcluster, "Resolution Out"=w340:string[][], "Func_ext 출력"=w339:string)  [unwired: 4 in]
      n123 = Index Array(array=w306) -> (element=w358:refnum<vi>)  [unwired: 1 in]
      n124 = call "Get Spec.vi"("NumRows"=w328, "Spec in"=w341, "Spec Ref."=w358, "error in"=w369, "Condition in"=w322, "Resolution in"=w340, "Func_ext"=w339) -> ("error out"=w370:errorcluster, "Data Out"=w364:string[][], "Func_ext Out"=w367:string)  [unwired: 2 out]
      n125 = call "Match_CMC.vi"("CMC IN"=w363, "error in"=w370, "Condition IN"=w364, "Func_ext"=w367) -> ("error out"=w346:errorcluster, "Func_ext out"=w366:string)  [unwired: 4 in, 2 out]
      n126 = case shown="\"10234-0\"" w336 {
        tunnel: w314 -> [w379 _ w389 _]
        tunnel: [w377 _ w386 _] -> w326
        tunnel: [w375 _ _ _] -> w325
        tunnel: [string[] ["채널", "Range"] string[] ["기준값", "단위"] string[] ["센서No."] _] -> w299
        frame "10223-0" {
          n127 = for {
            tunnel: w379 -> [w384] mode=indexing
            tunnel: [w380] -> w378 mode=indexing
            n128 = Index Array(array=w384) -> (element #1=w383:string, element #2=w382:string)  [unwired: 2 in]
            n129 = Format Into String(format string="%s_%s" ("포맷 문자열"), w383, w382) -> (resulting string=w380:string)  [unwired: 2 in, 1 out]
          }
          n130 = call-poly "Array Deduplication.vi"("배열 in"=w378) -> ("배열 out"=w377:string[])  [unwired: 9 in, 1 out]
          n131 = Build Array(w377) -> (w376:string[][])
          n132 = Transpose 2D Array(2D array=w376) -> (transposed array=w375:string[][])
        }
        frame "10227-0" {
        }
        frame "10234-0" {
          n133 = Index Array(array=w389, index (col)=0 ("비활성화된 인덱스 (열)")) -> (element=w387:string[])  [unwired: 1 in]
          n134 = call-poly "Array Deduplication.vi"("배열 in"=w387) -> ("배열 out"=w386:string[])  [unwired: 9 in, 1 out]
        }
        frame Default {
        }
      }
      n135 = Subtract(x=w313, y=2) -> (x-y=w324:i32)
      n136 = for {
        N: w324 -> [_]
        tunnel: [w391] -> w297 mode=indexing
        i -> [w394]
        n137 = Increment(x=w394) -> (x+1=w393:i32)
        n138 = Format Into String(format string="조건 %d" ("포맷 문자열"), w393) -> (resulting string=w391:string)  [unwired: 2 in, 1 out]
      }
      n139 = Empty Array?(array=w299) -> (empty?=w300:bool)
      n140 = Select(t=w297, s=w300, f=w299) -> (s? t:f=w298:string[])
      n141 = call "STD Cal Data.vi"("error in"=w346, "Data in"=w325, "Func_ext"=w366) -> ("error out"=w344:errorcluster, "Data Out"=w342:string[][], "Func_ext Out"=w320:string, "Data Out 2"=w343:string[])  [unwired: 4 in, 1 out]
      n142 = Build Array (concatenate)(w298, string[] ["명목값", "단위"]) -> (w327:string[])
      n143 = Index Array(array=w307) -> (element #1=w359:refnum<vi>, element #2=w354:refnum<vi>)  [unwired: 2 in]
      n144 = call-poly "Table Initialize.vi"("행의 개수"=w328, "Table Ref"=w359, "Value"=w314, "에러 입력"=w344, "열해더 문자열"=w327, "열의 개수"=w312) -> ("에러 출력"=w353:errorcluster, "Bottom"=w362:i32)  [unwired: 3 in, 1 out]
      n145 = call "Extract String.vi"("Resolution"=w301, "Condition"=w310) -> ("배열 1"=w311:string[], "배열 2"=w309:string[])  [unwired: 7 in, 1 out]
      n146 = property class="Tbl (엄격한)"(reference=w354, error in=w353, "Top"=w362, "Number of Rows"=w328) -> (reference out=w347:refnum<vi>, error out=w345:errorcluster)
      n147 = call-poly "Cell Spacing.vi"("Row Header in"=w361, "Col Header in"=w343, "error in"=w345, "Data in"=w342, "테이블 참조 in"=w347) -> ("error out"=w351:errorcluster)  [unwired: 4 in, 2 out]
      n148 = call "Meas2 status_1D Arr.vi"("행의 개수"=w328, "입력 클러스터"=w321, "행 헤더 문자열"=w326, "에러 입력"=w351, "Func_ext"=w320) -> ("에러 출력"=w305:errorcluster, "Func_ext Out"=w319:string)  [unwired: 5 in]
      n149 = call-poly "String Contents.vi"("문자 배열"=w309, "참조 배열"=w302, "에러 입력"=w305) -> ("에러 출력"=w304:errorcluster)  [unwired: 7 in, 1 out]
      n150 = call-poly "String Contents.vi"("문자 배열"=w311, "참조 배열"=w316, "에러 입력"=w304) -> ("에러 출력"=w317:errorcluster, "참조"=w315:refnum<vi>)  [unwired: 7 in]
      n151 = property on="표시형식" class="CmbBox"(reference=w315, error in=w317, "Strings[]"=w318) -> (error out=w303:errorcluster)  [unwired: 1 out]
      n152 = call "Certi Recall.vi"("큐 입력"=w348, "NumRows"=w328, "입력 클러스터"=w321, "에러 입력"=w303, "Func_ext in"=w319) -> ("에러 출력"=w349:errorcluster)  [unwired: 5 in, 1 out]
    }
    frame "Length_10" {
      n153 = Unbundle By Name(w512) -> ("Initialize 2.문자열"=w439:refnum<vi>[], "Initialize 2.테이블"=w476:refnum<vi>[], "Initialize 1.Condition"=w470:refnum<vi>[], "Initialize 1.Spec"=w469:refnum<vi>[], "Initialize 1.Resolution"=w495:refnum<vi>[], "Initialize 2.디지털(DBL)"=w457:refnum<vi>[], "Initialize 2.콤보박스"=w498:refnum<vi>[])
      n154 = call "Get Calproc.vi"("제목"=w509, "에러 입력"=w511, "Func_ext"=w510) -> ("에러 출력"=w468:errorcluster, "Condition"=w458:string[][], "Func_ext Out"=w479:string, "클러스터"=w492:T7)  [unwired: 5 in]
      n155 = Unbundle By Name(w492) -> ("Condition"=w453:string[][], "Spec"=w480:string[][], "CMC"=w484:string[][], "NumRows"=w462:u32)
      n156 = call "Variables Data IO.vi"("Select"=Cmd_Var_Data_IO."Condition Default", "error in"=w468, "Data In"=w458, "Func_ext"=w479) -> ("error out"=w467:errorcluster, "Func_ext Out"=w427:string)  [unwired: 5 in, 1 out]
      n157 = Index Array(array=w498) -> (element #1=w435:refnum<vi>, element #2=w431:refnum<vi>, element #3=w432:refnum<vi>)  [unwired: 3 in]
      n158 = property on="출력단위" class="CmbBox"(reference=w432, error in=w467) -> (error out=w497:errorcluster, "Value"=w463:string)  [unwired: 1 out]
      n159 = for {
        tunnel: w457 -> [w520] mode=indexing
        tunnel: [w516] -> w456 mode=indexing
        shift-right: [w519] -> w430
        shift-left: w497 -> [w518]
        tunnel: [w515] -> w454 mode=indexing
        n160 = property class="DigNum (엄격한)"(reference=w520, error in=w518) -> (error out=w519:errorcluster, "Value"=w516:dbl)  [unwired: 1 out]
        n161 = Format Into String(format string="%#f" ("포맷 문자열"), w516) -> (resulting string=w515:string)  [unwired: 2 in, 1 out]
      }
      n162 = call "Extract String.vi"("Condition"=w453) -> ("배열 2"=w459:string[], "측정범위"=w443:dbl[])  [unwired: 8 in, 1 out]
      n163 = Array Max & Min(array=w443) -> (max value=w507:dbl, min value=w504:dbl)  [unwired: 2 out]
      n164 = Index Array(array=w456) -> (element #1=w442:dbl, element #2=w440:dbl, element #3=w441:dbl)  [unwired: 3 in]
      n165 = Subtract(x=w443, y=w504) -> (x-y=w503:dbl[])
      n166 = Subtract(x=w507, y=w504) -> (x-y=w506:dbl)
      n167 = case shown="\"mV/V\"" w463 {
        selector: w463 -> [w526 w529 w532]
        tunnel: w442 -> [_ _ w537]
        tunnel: [w528 w531 w536] -> w499
        tunnel: w441 -> [w528 w531 w535]
        tunnel: ["0.00001" "0.0001" "0.0001"] -> w461
        tunnel: [w526 w529 "mV"] -> w496
        tunnel: [w526 w529 w532] -> w455
        frame Default {
        }
        frame "mA" {
        }
        frame "mV/V" {
          n168 = Multiply(x=w537, y=w535) -> (x*y=w536:dbl)
        }
      }
      n169 = property class="CmbBox"(reference=w431, error in=w430) -> (error out=w426:errorcluster, "Value"=w428:string)  [unwired: 1 out]
      n170 = Subtract(x=w499, y=w440) -> (x-y=w505:dbl)
      n171 = Divide(x=w506, y=w505) -> (x/y=w502:dbl)
      n172 = case shown="\"AC\"" w428 {
        tunnel: [T5."Disabled and Grayed Out" ("비활성화") T5."Enabled" ("비활성화")] -> w429
        frame "DC", Default {
        }
        frame "AC" {
        }
      }
      n173 = Divide(x=w503, y=w502) -> (x/y=w501:dbl[])
      n174 = Add(x=w501, y=w440) -> (x+y=w500:dbl[])
      n175 = Build Array (concatenate)(w454, w455) -> (w447:string[])
      n176 = Index Array(array=w495) -> (element=w494:refnum<vi>)  [unwired: 1 in]
      n177 = for {
        tunnel: w500 -> [w546] mode=indexing
        tunnel: w453 -> [w544] mode=indexing
        tunnel: [w542] -> w446 mode=indexing
        tunnel: w461 -> [w539]
        tunnel: w496 -> [w538]
        tunnel: [w540] -> w493 mode=indexing
        n178 = Format Into String(format string="%#f" ("포맷 문자열"), w546) -> (resulting string=w543:string)  [unwired: 2 in, 1 out]
        n179 = Build Array("Digital", w539, w538) -> (w540:string[])
        n180 = Insert Into Array(array=w544, new element #1=w543, new element #2=w538) -> (w542:string[])  [unwired: 1 in]
      }
      n181 = Index Array(array=w469) -> (element=w483:refnum<vi>)  [unwired: 1 in]
      n182 = Index Array(array=w470) -> (element=w508:refnum<vi>)  [unwired: 1 in]
      n183 = Index Array(array=w476) -> (element=w465:refnum<vi>)  [unwired: 1 in]
      n184 = Build Array (concatenate)(w459, w461) -> (w460:string[])
      n185 = call "Variables Data IO.vi"("Select"=Cmd_Var_Data_IO."Condition", "error in"=w426, "Data In"=w446, "Func_ext"=w427) -> ("error out"=w445:errorcluster, "Func_ext Out"=w420:string)  [unwired: 5 in, 1 out]
      n186 = call-poly "Table Initialize.vi"("행의 개수"=w462, "Table Ref"=w508, "Value"=w446, "에러 입력"=w445) -> ("에러 출력"=w474:errorcluster, "Bottom"=w473:i32)  [unwired: 5 in, 1 out]
      n187 = property class="Tbl (엄격한)"(reference=w465, error in=w474, "Top"=w473, "Number of Rows"=w462) -> (reference out=w444:refnum<vi>, error out=w424:errorcluster)
      n188 = Delete From Array(array=w439) -> (deleted portion=w437:refnum<vi>, array with subset deleted=w438:refnum<vi>[])  [unwired: 2 in]
      n189 = property class="CmbBox"(reference=w435, error in=w424, "DisabledEnum"=w429) -> (error out=w433:errorcluster, "Value"=w434:string)  [unwired: 1 out]
      n190 = for {
        tunnel: w446 -> [w521] mode=indexing
        tunnel: [w522] -> w472 mode=indexing
        n191 = Index Array(array=w521) -> (element #1=w525:string, element #2=w524:string)  [unwired: 2 in]
        n192 = Format Into String(format string="%s %s" ("포맷 문자열"), w525, w524) -> (resulting string=w522:string)  [unwired: 2 in, 1 out]
      }
      n193 = property class="Str"(reference=w437, error in=w433, "DisabledEnum"=w429) -> (error out=w422:errorcluster, "Value"=w436:string)  [unwired: 1 out]
      n194 = Build Array(w428, w436, w434) -> (w425:string[])
      n195 = Build Array(w447, w425) -> (w423:string[][])
      n196 = call "Variables Data IO.vi"("Select"=Cmd_Var_Data_IO."Condition_Temp", "error in"=w422, "Data In"=w423, "Func_ext"=w420) -> ("error out"=w421:errorcluster, "Func_ext Out"=w419:string)  [unwired: 5 in, 1 out]
      n197 = call "STD Cal Data.vi"("error in"=w421, "Data in"=w423, "Func_ext"=w419) -> ("error out"=w466:errorcluster, "Data Out"=w475:string[][], "Func_ext Out"=w448:string, "Data Out 2"=w471:string[])  [unwired: 4 in, 1 out]
      n198 = call-poly "Cell Spacing.vi"("Row Header in"=w472, "Col Header in"=w471, "error in"=w466, "Data in"=w475, "테이블 참조 in"=w444) -> ("error out"=w449:errorcluster)  [unwired: 4 in, 2 out]
      n199 = call "Create Resolution.vi"("행의 개수"=w462, "Table Ref"=w494, "에러 입력(에러 없음)"=w449, "Resolution"=w493, "Func_ext"=w448) -> ("에러 출력"=w481:errorcluster, "Resolution Out"=w482:string[][], "Func_ext 출력"=w489:string)  [unwired: 4 in]
      n200 = call "Get Spec.vi"("NumRows"=w462, "Spec in"=w480, "Spec Ref."=w483, "error in"=w481, "Condition in"=w446, "Resolution in"=w482, "Func_ext"=w489) -> ("error out"=w488:errorcluster, "Data Out"=w490:string[][], "Func_ext Out"=w491:string)  [unwired: 2 out]
      n201 = call "Match_CMC.vi"("CMC IN"=w484, "error in"=w488, "Condition IN"=w490, "Func_ext"=w491) -> ("error out"=w452:errorcluster, "Func_ext out"=w451:string)  [unwired: 4 in, 2 out]
      n202 = call-poly "String Contents.vi"("문자 배열"=w460, "참조 배열"=w438, "에러 입력"=w452) -> ("에러 출력"=w450:errorcluster)  [unwired: 7 in, 1 out]
      n203 = call "Certi Recall.vi"("큐 입력"=w486, "NumRows"=w462, "입력 클러스터"=w485, "에러 입력"=w450, "Func_ext in"=w451) -> ("에러 출력"=w487:errorcluster)  [unwired: 5 in, 1 out]
    }
    frame "Length_11" {
      n204 = Unbundle By Name(w600) -> ("Initialize 1.Measured"=w579:refnum<vi>[], "Initialize 1.Condition"=w597:refnum<vi>[], "Initialize 2.문자열"=w568:refnum<vi>[], "Initialize 1.Spec"=w574:refnum<vi>[])
      n205 = call "Get Calproc.vi"("제목"=w592, "에러 입력"=w606, "Func_ext"=w602) -> ("에러 출력"=w576:errorcluster, "Condition"=w549:string[][], "Func_ext Out"=w575:string, "클러스터"=w596:T7)  [unwired: 5 in]
      n206 = Unbundle By Name(w596) -> ("Spec"=w593:string[][], "CMC"=w591:string[][], "NumRows"=w571:u32, "Data"=w570:string[][])
      n207 = call "Variables Data IO.vi"("Select"=Cmd_Var_Data_IO."Condition Default", "error in"=w576, "Data In"=w549, "Func_ext"=w575) -> ("error out"=w577:errorcluster, "Func_ext Out"=w589:string)  [unwired: 5 in, 1 out]
      n208 = call "STD Cal Data.vi"("error in"=w577, "Func_ext"=w589) -> ("error out"=w583:errorcluster, "Data Out"=w580:string[][], "Func_ext Out"=w585:string)  [unwired: 5 in, 2 out]
      n209 = call "Create Resolution.vi"("에러 입력(에러 없음)"=w583, "Resolution"=w580, "Func_ext"=w585) -> ("에러 출력"=w582:errorcluster, "Resolution Out"=w581:string[][], "Func_ext 출력"=w584:string)  [unwired: 6 in]
      n210 = call "Extract String.vi"("Condition"=w549) -> ("배열 2"=w548:string[])  [unwired: 8 in, 2 out]
      n211 = Index Array(array=w580, index (row)=0 ("인덱스 (행)"), index (col)=1 ("비활성화된 인덱스 (열)")) -> (element=w586:string)
      n212 = Index Array(array=w574) -> (element=w553:refnum<vi>)  [unwired: 1 in]
      n213 = call "Get Spec.vi"("NumRows"=w571, "Spec in"=w593, "Spec Ref."=w553, "error in"=w582, "Condition in"=w549, "Resolution in"=w581, "Func_ext"=w584) -> ("error out"=w604:errorcluster, "Data Out"=w601:string[][], "Func_ext Out"=w603:string)  [unwired: 2 out]
      n214 = Build Array (concatenate)(w548, w586) -> (w599:string[])
      n215 = case shown="\"10228-2\"" w578 {
        tunnel: [w609 w613 string[] ["X-A", "X-B", "X-C", "Y-A", "Y-B", "Y-C"]] -> w562
        tunnel: [w608 w612 6] -> w560
        tunnel: w549 -> [w610 w617 w621]
        tunnel: [w610 w616 w621] -> w566
        tunnel: w570 -> [_ w619 _]
        tunnel: string[] ["1회", "2회", "3회", "4회", "5회"] -> [w609 w613 _]
        tunnel: 5 -> [w608 w612 _]
        tunnel: [w607 string[] ["형태", "명목값", "단위"] w620] -> w559
        tunnel: string[] ["명목값", "단위"] -> [w607 _ w620]
        frame Default {
        }
        frame "10229-0" {
          n216 = Index Array(array=w619, index (col)=6 ("비활성화된 인덱스 (열)")) -> (element=w615:string[])  [unwired: 1 in]
          n217 = Insert Into Array(array=w617, index (col)=0 ("비활성화된 인덱스 (열)"), new element=w615) -> (w616:string[][])  [unwired: 1 in]
        }
        frame "10228-2" {
        }
      }
      n218 = call "Match_CMC.vi"("CMC IN"=w591, "error in"=w604, "Condition IN"=w601, "Func_ext"=w603) -> ("error out"=w551:errorcluster, "Func_ext out"=w573:string)  [unwired: 4 in, 2 out]
      n219 = call-poly "String Contents.vi"("문자 배열"=w599, "참조 배열"=w568, "에러 입력"=w551) -> ("에러 출력"=w550:errorcluster)  [unwired: 7 in, 1 out]
      n220 = call "Variables Data IO.vi"("Select"=Cmd_Var_Data_IO."Condition", "error in"=w550, "Data In"=w566, "Func_ext"=w573) -> ("error out"=w572:errorcluster, "Func_ext Out"=w569:string)  [unwired: 5 in, 1 out]
      n221 = Array Size(array=w566) -> (size(s)=w565:i32[])
      n222 = Index Array(array=w597) -> (element=w554:refnum<vi>)  [unwired: 1 in]
      n223 = Index Array(array=w565) -> (element #2=w564:i32)  [unwired: 2 in, 1 out]
      n224 = Index Array(array=w579) -> (element=w552:refnum<vi>)  [unwired: 1 in]
      n225 = call-poly "Table Initialize.vi"("행의 개수"=w571, "Table Ref"=w554, "Value"=w566, "에러 입력"=w572, "열해더 문자열"=w559, "열의 개수"=w564) -> ("에러 출력"=w567:errorcluster)  [unwired: 3 in, 2 out]
      n226 = call-poly "Table Initialize.vi"("Table Ref"=w552, "에러 입력"=w567, "열해더 문자열"=w562, "열의 개수"=w560) -> ("에러 출력"=w557:errorcluster)  [unwired: 5 in, 2 out]
      n227 = Build Array(w554, w553, w552) -> (w547:refnum<vi>[])
      n228 = call "Tbl Comp.vi"("배열"=w547, "방향"=enum16{"수직", "수평"}."수평", "에러 입력"=w557) -> ("에러 출력"=w556:errorcluster)  [unwired: 6 in, 2 out]
      n229 = call "Certi Recall.vi"("큐 입력"=w594, "NumRows"=w571, "입력 클러스터"=w595, "에러 입력"=w556, "Func_ext in"=w569) -> ("에러 출력"=w590:errorcluster)  [unwired: 5 in, 1 out]
    }
    frame "Length_13" {
      n230 = Unbundle By Name(w689) -> ("Initialize 2.디지털(DBL)"=w635:refnum<vi>[], "Initialize 1.Spec"=w673:refnum<vi>[], "Initialize 2.콤보박스"=w665:refnum<vi>[], "Initialize 1.Condition"=w654:refnum<vi>[], "Initialize 2.문자열"=w655:refnum<vi>[])
      n231 = call "Get Calproc.vi"("제목"=w683, "에러 입력"=w694, "Func_ext"=w691) -> ("에러 출력"=w647:errorcluster, "Condition"=w646:string[][], "Func_ext Out"=w674:string, "클러스터"=w687:T7)  [unwired: 5 in]
      n232 = Unbundle By Name(w687) -> ("Data"=w652:string[][], "Spec"=w684:string[][], "CMC"=w682:string[][], "NumRows"=w672:u32)
      n233 = global read "Global_Cal STD.vi" "Cal STD"() -> (w662:string[][])
      n234 = Index Array(array=w655) -> (element #1=w656:refnum<vi>, element #2=w626:refnum<vi>, element #3=w625:refnum<vi>)  [unwired: 3 in]
      n235 = property class="Str"(reference=w625, error in=w647) -> (error out=w628:errorcluster, "Value"=w639:string)  [unwired: 1 out]
      n236 = call-poly "Data Classification.vi"("인덱스"=2, "DATA 입력"=w662, "검색 문자열"="Ring Gauge") -> ("DATA 출력"=w661:string[][])  [unwired: 4 in, 4 out]
      n237 = Index Array(array=w654) -> (element=w671:refnum<vi>)  [unwired: 1 in]
      n238 = for {
        tunnel: w652 -> [w713] mode=indexing
        tunnel: w639 -> [w708]
        tunnel: [w711] -> w629 mode=indexing
        tunnel: w646 -> [w710] mode=indexing
        tunnel: [w707] -> w645 mode=indexing
        n239 = Replace Array Subset(array=w710, new element=w708, index=0 ("인덱스")) -> (w707:string[])
        n240 = Replace Array Subset(array=w713, new element=w708, index=2 ("인덱스")) -> (w711:string[])
      }
      n241 = for {
        tunnel: w661 -> [w720] mode=indexing
        tunnel: [w714] -> w660 mode=indexing
        n242 = Index Array(array=w720, index #1=13 ("비활성화된 인덱스 (열)"), index #2=16 ("인덱스 (열)")) -> (element #1=w717:string, element #2=w715:string)
        n243 = Format Into String(format string="%s %s" ("포맷 문자열"), w717, w715) -> (resulting string=w714:string)  [unwired: 2 in, 1 out]
      }
      n244 = Index Array(array=w665) -> (element=w667:refnum<vi>)  [unwired: 1 in]
      n245 = Index Array(array=w673) -> (element #1=w670:refnum<vi>, element #2=w638:refnum<vi>)  [unwired: 2 in]
      n246 = call "Variables Data IO.vi"("Select"=Cmd_Var_Data_IO."Condition Default", "error in"=w628, "Data In"=w645, "Func_ext"=w674) -> ("error out"=w627:errorcluster, "Func_ext Out"=w651:string)  [unwired: 5 in, 1 out]
      n247 = Index Array(array=w635) -> (element=w634:refnum<vi>)  [unwired: 1 in]
      n248 = call "Variables Data IO.vi"("Select"=Cmd_Var_Data_IO."Condition", "error in"=w627, "Data In"=w629, "Func_ext"=w651) -> ("error out"=w653:errorcluster, "Func_ext Out"=w650:string)  [unwired: 5 in, 1 out]
      n249 = call-poly "Array Deduplication.vi"("배열 in"=w660) -> ("배열 out"=w659:string[])  [unwired: 9 in, 1 out]
      n250 = call-poly "Table Initialize.vi"("행의 개수"=w672, "Table Ref"=w671, "Value"=w629, "에러 입력"=w653) -> ("에러 출력"=w649:errorcluster)  [unwired: 5 in, 2 out]
      n251 = property class="CmbBox"(reference=w667, error in=w649, "Strings[]"=w659) -> (error out=w658:errorcluster, "Value"=w657:string)  [unwired: 1 out]
      n252 = call "STD Cal Data.vi"("error in"=w658, "문자열"=w657, "Func_ext"=w650) -> ("error out"=w642:errorcluster, "Data Out"=w675:string[][], "Func_ext Out"=w678:string, "Data Out 2"=w644:string[])  [unwired: 4 in, 1 out]
      n253 = Index Array(array=w644, index=15 ("인덱스")) -> (element=w640:string)
      n254 = property class="Str"(reference=w626, error in=w642, "Value"=w640) -> (error out=w641:errorcluster)  [unwired: 1 out]
      n255 = call "Create Resolution.vi"("에러 입력(에러 없음)"=w641, "Resolution"=w675, "Func_ext"=w678) -> ("에러 출력"=w668:errorcluster, "Resolution Out"=w676:string[][], "Func_ext 출력"=w677:string)  [unwired: 6 in]
      n256 = Index Array(array=w675, index (row)=0 ("인덱스 (행)"), index (col)=1 ("비활성화된 인덱스 (열)")) -> (element=w669:string)
      n257 = property class="Str"(reference=w656, error in=w668, "Value"=w669) -> (error out=w666:errorcluster)  [unwired: 1 out]
      n258 = call "Get Spec.vi"("NumRows"=w672, "Spec in"=w684, "Spec Ref."=w670, "error in"=w666, "Condition in"=w645, "Resolution in"=w676, "Func_ext"=w677) -> ("error out"=w637:errorcluster, "Data Out"=w690:string[][], "Spec Out"=w630:string[][], "Func_ext Out"=w692:string)  [unwired: 1 out]
      n259 = call "Match_CMC.vi"("CMC IN"=w682, "error in"=w637, "Condition IN"=w690, "Func_ext"=w692) -> ("error out"=w632:errorcluster, "Func_ext out"=w648:string)  [unwired: 4 in, 2 out]
      n260 = property class="DigNum (엄격한)"(reference=w634, error in=w632) -> (error out=w631:errorcluster, "Value"=w624:dbl)  [unwired: 1 out]
      n261 = for {
        tunnel: w630 -> [w697] mode=indexing
        tunnel: [w706] -> w633 mode=indexing
        tunnel: w624 -> [w699]
        n262 = Fract/Exp String To Number(string=w697) -> (number=w700:dbl[])  [unwired: 3 in, 1 out]
        n263 = Index Array(array=w697, index=0 ("비활성화된 인덱스 (열)")) -> (element=w695:string)
        n264 = call "Number Format.vi"("입력값"=w695) -> ("정밀도(단위적용)"=w701:i32)  [unwired: 10 in]
        n265 = Subtract(x=w700, y=w699) -> (x-y=w698:dbl[])
        n266 = Number To Fractional String(number=w698, precision (6)=w701) -> (F-format string=w705:string[])  [unwired: 2 in]
        n267 = Index Array(array=w705) -> (element #1=w704:string, element #2=w703:string)  [unwired: 2 in]
        n268 = Replace Array Subset(array=w697, new element #1=w704, index #1=0 ("인덱스"), new element #2=w703) -> (w706:string[])  [unwired: 1 in]
      }
      n269 = property class="Tbl (엄격한)"(reference=w638, error in=w631, "Value"=w633) -> (error out=w636:errorcluster)  [unwired: 1 out]
      n270 = call "Certi Recall.vi"("큐 입력"=w685, "NumRows"=w672, "입력 클러스터"=w686, "에러 입력"=w636, "Func_ext in"=w648) -> ("에러 출력"=w681:errorcluster)  [unwired: 5 in, 1 out]
    }
    frame "Length_14" {
      w724 = refnum<vi> refnum  # 라디오 버튼 컨트롤
      w785 = "Thread Plug Gauge Set" ("문자열 in")
      w784 = Cmd_File_path."데이터파일경로" ("항목")
      n271 = call "Get Calproc.vi"("제목"=w781, "에러 입력"=w798, "Func_ext"=w797) -> ("에러 출력"=w736:errorcluster, "Condition"=w780:string[][], "Func_ext Out"=w779:string, "클러스터"=w778:T7)  [unwired: 5 in]
      n272 = Unbundle By Name(w778) -> ("CMC"=w777:string[][], "Resolution"=w776:string[][], "NumRows"=w775:u32, "Spec"=w774:string[][])
      n273 = Unbundle By Name(w773) -> ("Initialize 2.ctrl"=w731:refnum<vi>[], "Initialize 2.문자열"=w735:refnum<vi>[], "Initialize 1.Resolution"=w772:refnum<vi>[], "Initialize 1.Condition"=w771:refnum<vi>[], "Initialize 2.열거형"=w770:refnum<vi>[])
      n274 = call "Variables Data IO.vi"("Select"=Cmd_Var_Data_IO."CMC Default", "error in"=w736, "Data In"=w777, "Func_ext"=w779) -> ("error out"=w751:errorcluster, "Func_ext Out"=w750:string)  [unwired: 5 in, 1 out]
      n275 = Index Array(array=w770) -> (element=w767:refnum<vi>)  [unwired: 1 in]
      n276 = property class="Enum"(reference=w767, error in=w751) -> (error out=w762:errorcluster, "Value"=w765:variant)  [unwired: 1 out]
      n277 = global read "Global_Cal Info.vi" "교정정보"() -> (w761:T9)
      n278 = global read "Global_Cal Info.vi" "기타정보"() -> (w760:cluster{"부서코드":string, "제조사코드":string})
      n279 = Unbundle By Name(w761) -> ("의뢰기관코드"=w759:string)
      n280 = Unbundle By Name(w760) -> ("부서코드"=w758:string)
      n281 = Variant To Data(error in=w762, type=0, Variant=w765) -> (data=w763:i32, error out=w766:errorcluster)
      n282 = for {
        tunnel: w771 -> [w821] mode=indexing
        shift-right: [w816] -> w748
        shift-left: w766 -> [w820]
        tunnel: w763 -> [w818]
        tunnel: w772 -> [w815] mode=indexing
        shift-right: [w813] -> w745
        shift-left: w750 -> [w814]
        tunnel: [w812] -> w740 mode=concatenating
        tunnel: w780 -> [w811]
        tunnel: w776 -> [w810]
        tunnel: w775 -> [w809]
        tunnel: w775 -> [w808]
        i -> [w819]
        n283 = case shown="기본" w818 {
          tunnel: w808 -> [w826 w836]
          tunnel: w821 -> [w825 w835]
          tunnel: w820 -> [w824 w834]
          tunnel: [w823 w833] -> w817
          tunnel: w811 -> [w822 w829]
          tunnel: w819 -> [_ w832]
          tunnel: [w822 w827] -> w812
          frame 0 {
            n284 = call-poly "Table Initialize.vi"("행의 개수"=w826, "Table Ref"=w825, "Value"=w822, "에러 입력"=w824) -> ("에러 출력"=w823:errorcluster)  [unwired: 5 in, 2 out]
          }
          frame Default {
            n285 = Equal?(x=w832, y=0) -> (x = y?=w830:bool)
            n286 = Select(t=w829, s=w830, f=string[][] []) -> (s? t:f=w827:string[][])
            n287 = call-poly "Table Initialize.vi"("행의 개수"=w836, "Table Ref"=w835, "Value"=w827, "에러 입력"=w834) -> ("에러 출력"=w833:errorcluster)  [unwired: 5 in, 2 out]
          }
        }
        n288 = call "Create Resolution.vi"("행의 개수"=w809, "Table Ref"=w815, "에러 입력(에러 없음)"=w817, "Resolution"=w810, "Func_ext"=w814) -> ("에러 출력"=w816:errorcluster, "Func_ext 출력"=w813:string)  [unwired: 4 in, 1 out]
      }
      n289 = Build Array(w759, w758) -> (w757:string[])
      n290 = for {
        tunnel: w757 -> [w803] mode=indexing
        shift-right: [w804] -> w755
        shift-left: w774 -> [w807]
        i -> [w801]
        n291 = Index Array(array=w807, index (col)=w801) -> (element=w806:string[])  [unwired: 1 in]
        n292 = Search 1D Array(1D array=w806, element=w803) -> (index of element=w805:i32)  [unwired: 1 in]
        n293 = Greater Or Equal To 0?(x=w805) -> (x >= 0?=w800:bool)
        n294 = Select(t=w803, s=w800, f="") -> (s? t:f=w802:string)
        n295 = call-poly "Data Classification.vi"("인덱스"=w801, "DATA 입력"=w807, "검색 문자열"=w802) -> ("DATA 출력"=w804:string[][])  [unwired: 4 in, 4 out]
      }
      n296 = Index Array(array=w735) -> (element=w734:refnum<vi>)  [unwired: 1 in]
      n297 = call "Variables Data IO.vi"("Select"=Cmd_Var_Data_IO."Condition", "error in"=w748, "Data In"=w740, "Func_ext"=w745) -> ("error out"=w747:errorcluster, "Func_ext Out"=w744:string)  [unwired: 5 in, 1 out]
      n298 = Array Subset(array=w740, index (col)=4 ("인덱스"), length (col)=2 ("길이")) -> (w737:string[][])  [unwired: 2 in]
      n299 = Delete From Array(array=w755, length=5 ("길이"), index (col)=0 ("비활성화된 인덱스 (열)")) -> (array with subset deleted=w754:string[][])  [unwired: 1 in, 1 out]
      n300 = call "Variables Data IO.vi"("Select"=Cmd_Var_Data_IO."Condition Default", "error in"=w747, "Data In"=w737, "Func_ext"=w744) -> ("error out"=w746:errorcluster, "Func_ext Out"=w743:string)  [unwired: 5 in, 1 out]
      n301 = call "Variables Data IO.vi"("Write blank data ?(F)"=TRUE ("Write blank data ?(T)"), "Select"=Cmd_Var_Data_IO."Spec Default", "error in"=w746, "Data In"=w754, "Func_ext"=w743) -> ("error out"=w733:errorcluster, "Func_ext Out"=w783:string)  [unwired: 4 in, 1 out]
      n302 = Index Array(array=w731) -> (element=w725:refnum<vi>)  [unwired: 1 in]
      n303 = property class="Str"(reference=w734, error in=w733, "Value"="" ("f")) -> (error out=w730:errorcluster)  [unwired: 1 out]
      n304 = To More Specific Class(target class=w724, reference=w725) -> (specific class reference=w723:refnum<vi>)  [unwired: 1 in, 1 out]
      n305 = property class="RadioBtnsControl"(reference=w723, error in=w730) -> (error out=w729:errorcluster, "Value"=w727:variant)  [unwired: 1 out]
      n306 = Variant To Data(error in=w729, type=enum32{"큰 값", "가까운 값"}."가까운 값" ("dw조건"), Variant=w727) -> (data=w722:enum32{"큰 값", "가까운 값"}, error out=w728:errorcluster)
      n307 = call "Create File Path.vi"("파일타입"=Cmd_File_Type."CSV", "항목"=w784, "문자열 in"=w785) -> ("파일경로"=w792:path)  [unwired: 5 in, 3 out]
      n308 = Format Into String(w722) -> (resulting string=w721:string)  [unwired: 3 in, 1 out]
      n309 = call-poly <vilib>:"Read Delimited Spreadsheet.vi"("file path (dialog if empty)"=w792, "delimiter (\\t)"="," ("delimiter (\\t)")) -> ("all rows"=w790:string[][])  [unwired: 8 in, 5 out]
      n310 = call "STD Cal Data.vi"("error in"=w728, "문자열"=w721, "Func_ext"=w783) -> ("error out"=w732:errorcluster, "Func_ext Out"=w782:string)  [unwired: 4 in, 3 out]
      n311 = call "Certi Recall.vi"("큐 입력"=w795, "NumRows"=w775, "입력 클러스터"=w796, "에러 입력"=w732, "Func_ext in"=w782) -> ("에러 출력"=w794:errorcluster)  [unwired: 5 in, 1 out]
      n312 = call "Create File Path.vi"("파일타입"=Cmd_File_Type."2진", "항목"=w784, "문자열 in"=w785) -> ("파일경로"=w788:path)  [unwired: 5 in, 3 out]
      n313 = Read from Binary File(5:string[][][] [], 11:w788) -> (2:w786:string[][][])  [unwired: 4 in, 3 out]
    }
    frame "Length_15" {
      n314 = call "Get Calproc.vi"("제목"=w877, "에러 입력"=w881, "Func_ext"=w880) -> ("에러 출력"=w876:errorcluster, "Condition"=w873:string[][], "Func_ext Out"=w869:string, "클러스터"=w878:T7)  [unwired: 5 in]
      n315 = Unbundle By Name(w879) -> ("Initialize 1.Spec"=w859:refnum<vi>[], "Initialize 2.콤보박스"=w868:refnum<vi>[], "Initialize 1.Condition"=w875:refnum<vi>[])
      n316 = Unbundle By Name(w878) -> ("Temp_1"=w872:string[][], "Spec"=w858:string[][], "CMC"=w854:string[][])
      n317 = call "Calcu_Surface Plate.vi"("Condition"=w873, "Data in"=w872) -> ("행크기"=w850:u32, "배열"=w837:string[][], "Data out"=w843:string[][])  [unwired: 7 in]
      n318 = Index Array(array=w875) -> (element=w874:refnum<vi>)  [unwired: 1 in]
      n319 = call-poly "Table Initialize.vi"("Table Ref"=w874, "Value"=w843, "에러 입력"=w876) -> ("에러 출력"=w870:errorcluster)  [unwired: 6 in, 2 out]
      n320 = call "Variables Data IO.vi"("Select"=Cmd_Var_Data_IO."Condition", "error in"=w870, "Data In"=w843, "Func_ext"=w869) -> ("error out"=w867:errorcluster, "Func_ext Out"=w861:string)  [unwired: 5 in, 1 out]
      n321 = Index Array(array=w868) -> (element=w866:refnum<vi>)  [unwired: 1 in]
      n322 = property class="CmbBox"(reference=w866, error in=w867) -> (error out=w862:errorcluster, "Value"=w865:string)  [unwired: 1 out]
      n323 = Build Array(w865, "˝" ("원소")) -> (w860:string[])
      n324 = Build Array(w860) -> (w844:string[][])
      n325 = call "Variables Data IO.vi"("Select"=Cmd_Var_Data_IO."Resolution", "error in"=w862, "Data In"=w844, "Func_ext"=w861) -> ("error out"=w839:errorcluster, "Func_ext Out"=w841:string)  [unwired: 5 in, 1 out]
      n326 = Index Array(array=w859) -> (element=w846:refnum<vi>)  [unwired: 1 in]
      n327 = call "Variables Data IO.vi"("Select"=Cmd_Var_Data_IO."Condition Default", "error in"=w839, "Data In"=w837, "Func_ext"=w841) -> ("error out"=w838:errorcluster, "Func_ext Out"=w840:string)  [unwired: 5 in, 1 out]
      n328 = call "Get Spec.vi"("NumRows"=w850, "Spec in"=w858, "Spec Ref."=w846, "error in"=w838, "Condition in"=w837, "Resolution in"=w837, "Func_ext"=w840) -> ("error out"=w856:errorcluster, "Data Out"=w855:string[][], "Func_ext Out"=w857:string)  [unwired: 2 out]
      n329 = call "Match_CMC.vi"("CMC IN"=w854, "error in"=w856, "Condition IN"=w855, "Func_ext"=w857) -> ("error out"=w853:errorcluster, "Func_ext out"=w849:string)  [unwired: 4 in, 2 out]
      n330 = call "STD Cal Data.vi"("error in"=w853, "Data in"=w844, "Func_ext"=w849) -> ("error out"=w845:errorcluster, "Func_ext Out"=w848:string)  [unwired: 4 in, 3 out]
      n331 = call "Certi Recall.vi"("Value"=w843, "큐 입력"=w852, "NumRows"=w850, "입력 클러스터"=w851, "에러 입력"=w845, "Func_ext in"=w848) -> ("에러 출력"=w847:errorcluster)  [unwired: 4 in, 1 out]
    }
    frame "Length_16" {
      n332 = Unbundle By Name(w931) -> ("Initialize 1.Condition"=w929:refnum<vi>[], "Initialize 1.Spec"=w917:refnum<vi>[], "Initialize 2.문자열"=w908:refnum<vi>[])
      n333 = call "Get Calproc.vi"("제목"=w925, "에러 입력"=w937, "Func_ext"=w933) -> ("에러 출력"=w906:errorcluster, "Condition"=w905:string[][], "Func_ext Out"=w918:string, "클러스터"=w928:T7)  [unwired: 5 in]
      n334 = Unbundle By Name(w928) -> ("Spec"=w891:string[][], "Data"=w884:string[][], "CMC"=w882:string[][], "NumRows"=w914:u32)
      n335 = Index Array(array=w908) -> (element #1=w889:refnum<vi>, element #2=w892:refnum<vi>, element #3=w894:refnum<vi>, element #4=w907:refnum<vi>)  [unwired: 4 in]
      n336 = property class="Str"(reference=w907, error in=w906) -> (error out=w902:errorcluster, "Value"=w904:string)  [unwired: 1 out]
      n337 = for {
        tunnel: w905 -> [w959] mode=indexing
        tunnel: w904 -> [w958]
        tunnel: [w957] -> w903 mode=indexing
        n338 = Replace Array Subset(array=w959, new element=w958) -> (w957:string[])  [unwired: 1 in]
      }
      n339 = call "Variables Data IO.vi"("Select"=Cmd_Var_Data_IO."Condition Default", "error in"=w902, "Data In"=w903, "Func_ext"=w918) -> ("error out"=w901:errorcluster, "Func_ext Out"=w923:string)  [unwired: 5 in, 1 out]
      n340 = call "STD Cal Data.vi"("error in"=w901, "Func_ext"=w923) -> ("error out"=w920:errorcluster, "Data Out"=w919:string[][], "Func_ext Out"=w922:string)  [unwired: 5 in, 2 out]
      n341 = call "Create Resolution.vi"("에러 입력(에러 없음)"=w920, "Resolution"=w919, "Func_ext"=w922) -> ("에러 출력"=w896:errorcluster, "Resolution Out"=w899:string[][], "Func_ext 출력"=w921:string)  [unwired: 6 in]
      n342 = Index Array(array=w917) -> (element=w910:refnum<vi>)  [unwired: 1 in]
      n343 = Index Array(array=w899, index (row)=0 ("인덱스 (행)"), index (col)=2 ("비활성화된 인덱스 (열)")) -> (element=w895:string)
      n344 = property class="Str"(reference=w894, error in=w896, "Value"=w895) -> (error out=w893:errorcluster)  [unwired: 1 out]
      n345 = Index Array(array=w929) -> (element=w911:refnum<vi>)  [unwired: 1 in]
      n346 = property class="Str"(reference=w892, error in=w893) -> (error out=w890:errorcluster, "Value"=w886:string)  [unwired: 1 out]
      n347 = property class="Str"(reference=w889, error in=w890) -> (error out=w888:errorcluster, "Value"=w887:string)  [unwired: 1 out]
      n348 = for {
        tunnel: w891 -> [w940] mode=indexing
        tunnel: w887 -> [w943]
        tunnel: w886 -> [w942]
        tunnel: [w941] -> w885 mode=indexing
        n349 = Index Array(array=w940, index=7 ("인덱스")) -> (element=w939:string)
        n350 = case shown="\"통과측\"" w939 {
          tunnel: w940 -> [w949 w950 w956]
          tunnel: w943 -> [_ _ w952]
          tunnel: w942 -> [w944 _ _]
          tunnel: [w947 w950 w954] -> w941
          frame "통과측" {
            n351 = Replace Array Subset(array=w949, new element #1=w944, index #1=20 ("인덱스"), new element #2="0" ("새 원소/부분배열"), new element #3="mm" ("새 원소/부분배열")) -> (w947:string[])  [unwired: 2 in]
          }
          frame Default {
          }
          frame "정지측" {
            n352 = Replace Array Subset(array=w956, new element #1="0" ("새 원소/부분배열"), index #1=20 ("인덱스"), new element #2=w952, new element #3="mm" ("새 원소/부분배열")) -> (w954:string[])  [unwired: 2 in]
          }
        }
      }
      n353 = Insert Into Array(array=w903, index (col)=0 ("비활성화된 인덱스 (열)"), new element=w884) -> (w883:string[][])  [unwired: 1 in]
      n354 = call "Get Spec.vi"("NumRows"=w914, "Spec in"=w885, "Spec Ref."=w910, "error in"=w888, "Condition in"=w883, "Resolution in"=w899, "Func_ext"=w921) -> ("error out"=w935:errorcluster, "Data Out"=w932:string[][], "Func_ext Out"=w934:string)  [unwired: 2 out]
      n355 = call "Match_CMC.vi"("CMC IN"=w882, "error in"=w935, "Condition IN"=w932, "Func_ext"=w934) -> ("error out"=w900:errorcluster, "Func_ext out"=w916:string)  [unwired: 4 in, 2 out]
      n356 = call "Variables Data IO.vi"("Select"=Cmd_Var_Data_IO."Condition", "error in"=w900, "Data In"=w883, "Func_ext"=w916) -> ("error out"=w915:errorcluster, "Func_ext Out"=w913:string)  [unwired: 5 in, 1 out]
      n357 = call-poly "Table Initialize.vi"("행의 개수"=w914, "Table Ref"=w911, "Value"=w883, "에러 입력"=w915) -> ("에러 출력"=w912:errorcluster)  [unwired: 5 in, 2 out]
      n358 = call "Certi Recall.vi"("큐 입력"=w926, "NumRows"=w914, "입력 클러스터"=w927, "에러 입력"=w912, "Func_ext in"=w913) -> ("에러 출력"=w924:errorcluster)  [unwired: 5 in, 1 out]
    }
    frame "Length_2" {
      n359 = Unbundle By Name(w1022) -> ("Initialize 1.Condition"=w995:refnum<vi>[], "Initialize 2.콤보박스"=w972:refnum<vi>[], "Initialize 2.문자열"=w975:refnum<vi>[], "Initialize 1.Spec"=w974:refnum<vi>[], "Initialize 1.Resolution"=w979:refnum<vi>[])
      n360 = call "Get Calproc.vi"("제목"=w1006, "에러 입력"=w1030, "Func_ext"=w1026) -> ("에러 출력"=w984:errorcluster, "Func_ext Out"=w983:string, "클러스터"=w1013:T7)  [unwired: 5 in, 1 out]
      n361 = Unbundle By Name(w1013) -> ("Temp_1"=w985:string[][], "NumRows"=w980:u32, "Condition"=w965:string[][], "Resolution"=w960:string[][], "Spec"=w1009:string[][], "CMC"=w1024:string[][], "Data"=w1002:string[][], "Temp_1"=w986:string[][])
      n362 = call "Array Size.vi"("Data in"=w986) -> ("열(I32)"=w1001:i32)  [unwired: 7 in, 3 out]
      n363 = call "Variables Data IO.vi"("Select"=Cmd_Var_Data_IO."Condition_Temp", "error in"=w984, "Data In"=w985, "Func_ext"=w983) -> ("error out"=w981:errorcluster, "Func_ext Out"=w982:string)  [unwired: 5 in, 1 out]
      n364 = call "Variables Data IO.vi"("Select"=Cmd_Var_Data_IO."Condition Default", "error in"=w981, "Data In"=w965, "Func_ext"=w982) -> ("error out"=w973:errorcluster, "Func_ext Out"=w978:string)  [unwired: 5 in, 1 out]
      n365 = case shown="기본" w1001 {
        tunnel: w1002 -> [w1033 w1041]
        tunnel: [w1032 w1040] -> w1023
        frame 1 {
          n366 = for {
            tunnel: w1033 -> [w1039] mode=indexing
            tunnel: [w1034] -> w1032 mode=indexing
            n367 = Index Array(array=w1039) -> (element #1=w1038:string, element #2=w1037:string, element #3=w1036:string)  [unwired: 3 in]
            n368 = Format Into String(format string="%s (%s %s)" ("포맷 문자열"), w1038, w1037, w1036) -> (resulting string=w1034:string)  [unwired: 2 in, 1 out]
          }
        }
        frame Default {
          n369 = for {
            tunnel: w1041 -> [w1046] mode=indexing
            tunnel: [w1042] -> w1040 mode=indexing
            n370 = Index Array(array=w1046) -> (element #1=w1045:string, element #2=w1044:string)  [unwired: 2 in]
            n371 = Format Into String(format string="%s %s" ("포맷 문자열"), w1045, w1044) -> (resulting string=w1042:string)  [unwired: 2 in, 1 out]
          }
        }
      }
      n372 = Index Array(array=w979) -> (element=w1007:refnum<vi>)  [unwired: 1 in]
      n373 = call "Create Resolution.vi"("행의 개수"=w980, "Table Ref"=w1007, "에러 입력(에러 없음)"=w973, "Resolution"=w960, "Func_ext"=w978) -> ("에러 출력"=w976:errorcluster, "Resolution Out"=w1008:string[][], "Func_ext 출력"=w977:string)  [unwired: 4 in]
      n374 = Index Array(array=w974) -> (element=w1020:refnum<vi>)  [unwired: 1 in]
      n375 = call "Get Spec.vi"("NumRows"=w980, "Spec in"=w1009, "Spec Ref."=w1020, "error in"=w976, "Condition in"=w965, "Resolution in"=w1008, "Func_ext"=w977) -> ("error out"=w997:errorcluster, "Data Out"=w1025:string[][], "Func_ext Out"=w1027:string)  [unwired: 2 out]
      n376 = Index Array(array=w975) -> (element #1=w1000:refnum<vi>, element #2=w999:refnum<vi>)  [unwired: 2 in]
      n377 = call "Match_CMC.vi"("CMC IN"=w1024, "error in"=w997, "Condition IN"=w1025, "Func_ext"=w1027) -> ("error out"=w994:errorcluster, "Func_ext out"=w996:string)  [unwired: 4 in, 2 out]
      n378 = Build Array(w1000, w999, w999) -> (w998:refnum<vi>[])
      n379 = Add(x=2 ("y"), y=w1001) -> (x+y=w1018:i32)
      n380 = call "Variables Data IO.vi"("Select"=Cmd_Var_Data_IO."Condition", "error in"=w994, "Data In"=w1002, "Func_ext"=w996) -> ("error out"=w963:errorcluster, "Func_ext Out"=w971:string)  [unwired: 5 in, 1 out]
      n381 = for {
        N: w1001 -> [_]
        tunnel: [""] -> w1017 mode=indexing
      }
      n382 = call "Extract String.vi"("Resolution"=w960, "Condition"=w965) -> ("배열 1"=w966:string[], "배열 2"=w964:string[])  [unwired: 7 in, 1 out]
      n383 = To Unsigned Long Integer(number=w1018) -> (unsigned 32bit integer=w1019:u32)
      n384 = call-poly "String Contents.vi"("문자 배열"=w964, "참조 배열"=w998, "에러 입력"=w963) -> ("에러 출력"=w962:errorcluster)  [unwired: 7 in, 1 out]
      n385 = Build Array (concatenate)(w1017, string[] ["명목값", "단위"]) -> (w1015:string[])
      n386 = call-poly "String Contents.vi"("문자 배열"=w966, "참조 배열"=w972, "에러 입력"=w962) -> ("에러 출력"=w961:errorcluster)  [unwired: 7 in, 1 out]
      n387 = Index Array(array=w995) -> (element #1=w989:refnum<vi>, element #2=w993:refnum<vi>)  [unwired: 2 in]
      n388 = call-poly "Table Initialize.vi"("행의 개수"=w980, "Table Ref"=w989, "Value"=w1002, "에러 입력"=w961) -> ("에러 출력"=w987:errorcluster, "Bottom"=w967:i32, "Table Ref out"=w988:refnum<vi>)  [unwired: 5 in]
      n389 = property on="Condition" class="Tbl"(reference=w988, error in=w987, "Number of Columns"=w1019, "Column Headers[]"=w1015) -> (error out=w970:errorcluster)  [unwired: 1 out]
      n390 = call "STD Cal Data.vi"("error in"=w970, "Func_ext"=w971) -> ("error out"=w991:errorcluster, "Data Out"=w1010:string[][], "Func_ext Out"=w1004:string)  [unwired: 5 in, 2 out]
      n391 = call-poly "Cell Spacing.vi"("Row Header in"=w1023, "error in"=w991, "Data in"=w1010, "테이블 참조 in"=w993) -> ("error out"=w990:errorcluster, "테이블 참조 Out"=w992:refnum<vi>)  [unwired: 5 in, 1 out]
      n392 = property class="Tbl"(reference=w992, error in=w990, "Top"=w967, "Number of Rows"=w980) -> (error out=w969:errorcluster)  [unwired: 1 out]
      n393 = call "Meas2 status_1D Arr.vi"("입력 클러스터"=w1005, "에러 입력"=w969, "Func_ext"=w1004) -> ("에러 출력"=w968:errorcluster, "Func_ext Out"=w1003:string)  [unwired: 7 in]
      n394 = call "Certi Recall.vi"("큐 입력"=w1011, "NumRows"=w980, "입력 클러스터"=w1005, "에러 입력"=w968, "Func_ext in"=w1003) -> ("에러 출력"=w1012:errorcluster)  [unwired: 5 in, 1 out]
    }
    frame "Length_3" {
      w1089 = string[] ["명목값", "기준값", "단위"] ("열 헤더 문자열[]")
      w1083 = 0 ("인덱스 (행)")
      n395 = Unbundle By Name(w1086) -> ("Initialize 1.Measured"=w1049:refnum<vi>[], "Initialize 2.콤보박스"=w1061:refnum<vi>[], "Initialize 2.문자열"=w1085:refnum<vi>[], "Initialize 1.Condition"=w1071:refnum<vi>[], "Initialize 1.Spec"=w1069:refnum<vi>[], "Initialize 1.Resolution"=w1070:refnum<vi>[])
      n396 = call "Get Calproc.vi"("제목"=w1072, "에러 입력"=w1109, "Func_ext"=w1102) -> ("에러 출력"=w1108:errorcluster, "Condition"=w1068:string[][], "Func_ext Out"=w1103:string, "클러스터"=w1082:T7)  [unwired: 5 in]
      n397 = Unbundle By Name(w1082) -> ("Resolution"=w1067:string[][], "Spec"=w1077:string[][], "CMC"=w1100:string[][], "NumRows"=w1073:u32, "Condition"=w1064:string[][], "Resolution"=w1063:string[][], "Temp_1"=w1047:string[][])
      n398 = Index Array(array=w1047, index (row)=w1083, index (col)=w1083) -> (element=w1057:string)
      n399 = call "Variables Data IO.vi"("Select"=Cmd_Var_Data_IO."Condition Default", "error in"=w1108, "Data In"=w1068, "Func_ext"=w1103) -> ("error out"=w1098:errorcluster, "Func_ext Out"=w1099:string)  [unwired: 5 in, 1 out]
      n400 = call "Extract String.vi"("Resolution"=w1063, "Condition"=w1064) -> ("배열 1"=w1059:string[], "배열 2"=w1062:string[])  [unwired: 7 in, 1 out]
      n401 = Build Array (concatenate)(w1059, w1057) -> (w1058:string[])
      n402 = call "STD Cal Data.vi"("error in"=w1098, "Data in"=w1047, "Func_ext"=w1099) -> ("error out"=w1096:errorcluster, "Data Out"=w1065:string[][], "Func_ext Out"=w1095:string)  [unwired: 4 in, 2 out]
      n403 = Index Array(array=w1070) -> (element=w1074:refnum<vi>)  [unwired: 1 in]
      n404 = call "Variables Data IO.vi"("Select"=Cmd_Var_Data_IO."Condition", "error in"=w1096, "Data In"=w1065, "Func_ext"=w1095) -> ("error out"=w1093:errorcluster, "Func_ext Out"=w1094:string)  [unwired: 5 in, 1 out]
      n405 = Index Array(array=w1069) -> (element=w1087:refnum<vi>)  [unwired: 1 in]
      n406 = call "Create Resolution.vi"("행의 개수"=w1073, "Table Ref"=w1074, "에러 입력(에러 없음)"=w1093, "Resolution"=w1067, "Func_ext"=w1094) -> ("에러 출력"=w1105:errorcluster, "Resolution Out"=w1076:string[][], "Func_ext 출력"=w1075:string)  [unwired: 4 in]
      n407 = Index Array(array=w1071) -> (element=w1090:refnum<vi>)  [unwired: 1 in]
      n408 = call "Get Spec.vi"("NumRows"=w1073, "Spec in"=w1077, "Spec Ref."=w1087, "error in"=w1105, "Condition in"=w1065, "Resolution in"=w1076, "Func_ext"=w1075) -> ("error out"=w1106:errorcluster, "Data Out"=w1101:string[][], "Func_ext Out"=w1104:string)  [unwired: 2 out]
      n409 = call "Match_CMC.vi"("CMC IN"=w1100, "error in"=w1106, "Condition IN"=w1101, "Func_ext"=w1104) -> ("error out"=w1092:errorcluster, "Func_ext out"=w1051:string)  [unwired: 4 in, 2 out]
      n410 = Array Size(array=w1089) -> (size(s)=w1088:i32)
      n411 = call-poly "Table Initialize.vi"("행의 개수"=w1073, "Table Ref"=w1090, "Value"=w1065, "에러 입력"=w1092) -> ("에러 출력"=w1091:errorcluster, "Table Ref out"=w1066:refnum<vi>)  [unwired: 5 in, 1 out]
      n412 = To Unsigned Long Integer(number=w1088) -> (unsigned 32bit integer=w1056:u32)
      n413 = property on="Condition" class="Tbl"(reference=w1066, error in=w1091, "Column Headers[]"=w1089, "Number of Columns"=w1056) -> (error out=w1084:errorcluster)  [unwired: 1 out]
      n414 = call-poly "String Contents.vi"("문자 배열"=w1062, "참조 배열"=w1085, "에러 입력"=w1084) -> ("에러 출력"=w1060:errorcluster)  [unwired: 7 in, 1 out]
      n415 = call-poly "String Contents.vi"("문자 배열"=w1058, "참조 배열"=w1061, "에러 입력"=w1060) -> ("에러 출력"=w1054:errorcluster)  [unwired: 7 in, 1 out]
      n416 = Delete From Array(array=w1049) -> (array with subset deleted=w1048:refnum<vi>[])  [unwired: 2 in, 1 out]
      n417 = Build Array (concatenate)(w1071, w1070, w1069, w1048) -> (w1055:refnum<vi>[])
      n418 = call "Meas2 status_1D Arr.vi"("입력 클러스터"=w1052, "에러 입력"=w1054, "Func_ext"=w1051) -> ("에러 출력"=w1053:errorcluster, "Func_ext Out"=w1050:string)  [unwired: 7 in]
      n419 = call "Tbl Comp.vi"("배열"=w1055, "방향"=enum16{"수직", "수평"}."수평", "에러 입력"=w1053) -> ("에러 출력"=w1081:errorcluster)  [unwired: 6 in, 2 out]
      n420 = call "Certi Recall.vi"("큐 입력"=w1079, "NumRows"=w1073, "입력 클러스터"=w1052, "에러 입력"=w1081, "Func_ext in"=w1050) -> ("에러 출력"=w1080:errorcluster)  [unwired: 5 in, 1 out]
    }
    frame "Length_4" {
      n421 = Unbundle By Name(w1161) -> ("Initialize 1.Condition"=w1120:refnum<vi>[], "Initialize 1.Spec"=w1122:refnum<vi>[], "Initialize 1.Measured"=w1146:refnum<vi>[], "Initialize 2.콤보박스"=w1126:refnum<vi>[], "Initialize 2.문자열"=w1127:refnum<vi>[], "Initialize 1.Spec"=w1121:refnum<vi>[], "Initialize 1.Condition"=w1123:refnum<vi>[])
      n422 = call "Get Calproc.vi"("제목"=w1139, "에러 입력"=w1168, "Func_ext"=w1164) -> ("에러 출력"=w1124:errorcluster, "Condition"=w1136:string[][], "Func_ext Out"=w1128:string, "클러스터"=w1149:T7)  [unwired: 5 in]
      n423 = Unbundle By Name(w1149) -> ("Temp_1"=w1137:string[][], "Spec"=w1140:string[][], "NumRows"=w1141:u32, "CMC"=w1138:string[][], "Resolution"=w1131:string[][], "Condition"=w1125:string[][])
      n424 = call "Variables Data IO.vi"("Select"=Cmd_Var_Data_IO."Condition", "error in"=w1124, "Data In"=w1136, "Func_ext"=w1128) -> ("error out"=w1145:errorcluster, "Func_ext Out"=w1144:string)  [unwired: 5 in, 1 out]
      n425 = call "Variables Data IO.vi"("Select"=Cmd_Var_Data_IO."Condition Default", "error in"=w1145, "Data In"=w1136, "Func_ext"=w1144) -> ("error out"=w1143:errorcluster, "Func_ext Out"=w1129:string)  [unwired: 5 in, 1 out]
      n426 = Index Array(array=w1123) -> (element=w1159:refnum<vi>)  [unwired: 1 in]
      n427 = call "Extract String.vi"("Condition"=w1125) -> ("배열 1"=w1133:string[], "배열 2"=w1135:string[])  [unwired: 8 in, 1 out]
      n428 = call-poly "Table Initialize.vi"("행의 개수"=w1141, "Table Ref"=w1159, "Value"=w1136, "에러 입력"=w1143) -> ("에러 출력"=w1130:errorcluster)  [unwired: 5 in, 2 out]
      n429 = Index Array(array=w1121) -> (element=w1162:refnum<vi>)  [unwired: 1 in]
      n430 = call "Get Spec.vi"("NumRows"=w1141, "Spec in"=w1140, "Spec Ref."=w1162, "error in"=w1130, "Condition in"=w1136, "Resolution in"=w1137, "Func_ext"=w1129) -> ("error out"=w1166:errorcluster, "Data Out"=w1163:string[][], "Func_ext Out"=w1165:string)  [unwired: 2 out]
      n431 = call "Match_CMC.vi"("CMC IN"=w1138, "error in"=w1166, "Condition IN"=w1163, "Func_ext"=w1165) -> ("error out"=w1119:errorcluster, "Func_ext out"=w1132:string)  [unwired: 4 in, 2 out]
      n432 = call "Variables Data IO.vi"("Select"=Cmd_Var_Data_IO."Resolution", "error in"=w1119, "Data In"=w1131, "Func_ext"=w1132) -> ("error out"=w1118:errorcluster, "Func_ext Out"=w1112:string)  [unwired: 5 in, 1 out]
      n433 = call "STD Cal Data.vi"("error in"=w1118, "Func_ext"=w1112) -> ("error out"=w1117:errorcluster, "Func_ext Out"=w1111:string, "Cal STD"=w1158:string[][])  [unwired: 5 in, 2 out]
      n434 = Index Array(array=w1158, index (col)=28 ("비활성화된 인덱스 (열)")) -> (element=w1155:string[])  [unwired: 1 in]
      n435 = call-poly "Array Deduplication.vi"("배열 in"=w1155) -> ("배열 out"=w1154:string[])  [unwired: 9 in, 1 out]
      n436 = Build Array (concatenate)(w1120, w1122, w1146) -> (w1110:refnum<vi>[])
      n437 = for {
        tunnel: w1154 -> [w1175]
        tunnel: string[] ["2", "1", "0", "K"] -> [w1172] mode=indexing
        tunnel: [w1172] -> w1151
        stop <- w1173 stop-if-true
        n438 = Search 1D Array(1D array=w1175, element=w1172) -> (index of element=w1174:i32)  [unwired: 1 in]
        n439 = Greater Or Equal To 0?(x=w1174) -> (x >= 0?=w1173:bool)
      }
      n440 = case shown="\"0\"" w1151 {
        tunnel: [cluster{"String":string, "Value":string}[] [{"String"="0급", "Value"="0급"}, {"String"="1급", "Value"="1급"}, {"String"="2급 또는 확인불가", "Value"="2급"}] ("문자열과 값[]") cluster{"String":string, "Value":string}[] [{"String"="1급", "Value"="1급"}, {"String"="2급 또는 확인불가", "Value"="2급"}] ("문자열과 값[]") cluster{"String":string, "Value":string}[] [{"String"="2급 또는 확인불가", "Value"="2급"}] ("문자열과 값[]") _] -> w1150
        frame Default {
        }
        frame "0" {
        }
        frame "1" {
        }
        frame "2" {
        }
      }
      n441 = Index Array(array=w1126) -> (element=w1152:refnum<vi>)  [unwired: 1 in]
      n442 = property class="CmbBox"(reference=w1152, error in=w1117, "Strings And Values[]"=w1150) -> (error out=w1116:errorcluster)  [unwired: 1 out]
      n443 = call-poly "String Contents.vi"("문자 배열"=w1135, "참조 배열"=w1127, "에러 입력"=w1116) -> ("에러 출력"=w1134:errorcluster)  [unwired: 7 in, 1 out]
      n444 = call-poly "String Contents.vi"("문자 배열"=w1133, "참조 배열"=w1126, "에러 입력"=w1134) -> ("에러 출력"=w1115:errorcluster)  [unwired: 7 in, 1 out]
      n445 = call "Tbl Comp.vi"("배열"=w1110, "방향"=enum16{"수직", "수평"}."수평", "에러 입력"=w1115) -> ("에러 출력"=w1114:errorcluster)  [unwired: 6 in, 2 out]
      n446 = call "Certi Recall.vi"("큐 입력"=w1147, "NumRows"=w1141, "입력 클러스터"=w1148, "에러 입력"=w1114, "Func_ext in"=w1111) -> ("에러 출력"=w1113:errorcluster)  [unwired: 5 in, 1 out]
    }
    frame "Length_5" {
      n447 = Unbundle By Name(w1229) -> ("Initialize 2.콤보박스"=w1212:refnum<vi>[], "Initialize 2.문자열"=w1184:refnum<vi>[], "Initialize 1.Condition"=w1219:refnum<vi>[], "Initialize 1.Spec"=w1231:refnum<vi>[], "Initialize 1.Resolution"=w1220:refnum<vi>[], "Initialize 1.Measured"=w1195:refnum<vi>[], "Initialize 1.Measured_ADJ"=w1196:refnum<vi>[])
      n448 = call "Get Calproc.vi"("제목"=w1214, "에러 입력"=w1239, "Func_ext"=w1233) -> ("에러 출력"=w1238:errorcluster, "Condition"=w1209:string[][], "Func_ext Out"=w1234:string, "클러스터"=w1227:T7)  [unwired: 5 in]
      n449 = Unbundle By Name(w1227) -> ("Data"=w1208:string[][], "제목"=w1176:string, "Resolution"=w1200:string[][], "Spec"=w1218:string[][], "CMC"=w1230:string[][], "NumRows"=w1191:u32)
      n450 = call "Variables Data IO.vi"("Select"=Cmd_Var_Data_IO."Condition Default", "error in"=w1238, "Data In"=w1209, "Func_ext"=w1234) -> ("error out"=w1223:errorcluster, "Func_ext Out"=w1222:string)  [unwired: 5 in, 1 out]
      n451 = case shown="\"10511-3\"" w1187 {
        tunnel: w1200 -> [w1242 w1244 w1253]
        tunnel: [w1242 w1244 w1254] -> w1211
        tunnel: w1209 -> [w1241 w1249 w1252]
        tunnel: [w1241 w1248 w1252] -> w1201
        tunnel: w1208 -> [_ w1245 _]
        tunnel: [w1240 string[] ["명목값", "단위", "배율"] w1251] -> w1203
        tunnel: string[] ["명목값", "단위"] -> [w1240 _ w1251]
        frame Default {
        }
        frame "10511-3" {
          n452 = Index Array(array=w1245, index (col)=5 ("비활성화된 인덱스 (열)")) -> (element=w1247:string[])  [unwired: 1 in]
          n453 = Insert Into Array(array=w1249, index (col)=2 ("비활성화된 인덱스 (열)"), new element=w1247) -> (w1248:string[][])  [unwired: 1 in]
        }
        frame "10233-0" {
          n454 = for {
            tunnel: [w1255] -> w1254 mode=indexing
            tunnel: w1253 -> [_] mode=indexing
            n455 = Build Array("Digital", "0.001" ("원소"), "mm" ("원소")) -> (w1255:string[])
          }
        }
      }
      n456 = Index Array(array=w1220) -> (element=w1205:refnum<vi>)  [unwired: 1 in]
      n457 = call "Variables Data IO.vi"("Select"=Cmd_Var_Data_IO."Condition", "error in"=w1223, "Data In"=w1201, "Func_ext"=w1222) -> ("error out"=w1189:errorcluster, "Func_ext Out"=w1188:string)  [unwired: 5 in, 1 out]
      n458 = Index Array(array=w1231) -> (element=w1204:refnum<vi>)  [unwired: 1 in]
      n459 = call "Create Resolution.vi"("행의 개수"=w1191, "Table Ref"=w1205, "에러 입력(에러 없음)"=w1189, "Resolution"=w1211, "Func_ext"=w1188) -> ("에러 출력"=w1216:errorcluster, "Resolution Out"=w1217:string[][], "Func_ext 출력"=w1215:string)  [unwired: 4 in]
      n460 = Index Array(array=w1219) -> (element=w1206:refnum<vi>)  [unwired: 1 in]
      n461 = call "Get Spec.vi"("NumRows"=w1191, "Spec in"=w1218, "Spec Ref."=w1204, "error in"=w1216, "Condition in"=w1201, "Resolution in"=w1217, "Func_ext"=w1215) -> ("error out"=w1236:errorcluster, "Data Out"=w1232:string[][], "Func_ext Out"=w1235:string)  [unwired: 2 out]
      n462 = call "Match_CMC.vi"("CMC IN"=w1230, "error in"=w1236, "Condition IN"=w1232, "Func_ext"=w1235) -> ("error out"=w1228:errorcluster, "Func_ext out"=w1192:string)  [unwired: 4 in, 2 out]
      n463 = call-poly "Table Initialize.vi"("행의 개수"=w1191, "Table Ref"=w1206, "Value"=w1201, "에러 입력"=w1228, "열해더 문자열"=w1203) -> ("에러 출력"=w1194:errorcluster)  [unwired: 4 in, 2 out]
      n464 = call "Meas2 status_1D Arr.vi"("행의 개수"=w1191, "입력 클러스터"=w1190, "에러 입력"=w1194, "Func_ext"=w1192) -> ("에러 출력"=w1193:errorcluster, "Func_ext Out"=w1186:string)  [unwired: 6 in]
      n465 = Build Array (concatenate)(w1206, w1205, w1204, w1195, w1196) -> (w1197:refnum<vi>[])
      n466 = call "Tbl Comp.vi"("배열"=w1197, "방향"=enum16{"수직", "수평"}."수평", "에러 입력"=w1193) -> ("에러 출력"=w1183:errorcluster)  [unwired: 6 in, 2 out]
      n467 = call "Extract String.vi"("Resolution"=w1200, "Condition"=w1201) -> ("배열 1"=w1199:string[], "배열 2"=w1180:string[])  [unwired: 7 in, 1 out]
      n468 = call "STD Cal Data.vi"("error in"=w1183, "문자열"=w1176, "Func_ext"=w1186) -> ("error out"=w1181:errorcluster, "Func_ext Out"=w1185:string, "Data Out 2"=w1178:string[])  [unwired: 4 in, 2 out]
      n469 = Index Array(array=w1178) -> (element=w1177:string)  [unwired: 1 in]
      n470 = Insert Into Array(array=w1180, new element=w1177) -> (w1179:string[])  [unwired: 1 in]
      n471 = call-poly "String Contents.vi"("문자 배열"=w1179, "참조 배열"=w1184, "에러 입력"=w1181) -> ("에러 출력"=w1182:errorcluster)  [unwired: 7 in, 1 out]
      n472 = call-poly "String Contents.vi"("문자 배열"=w1199, "참조 배열"=w1212, "에러 입력"=w1182) -> ("에러 출력"=w1213:errorcluster, "참조"=w1198:refnum<vi>)  [unwired: 7 in]
      n473 = property on="표시형식" class="CmbBox"(reference=w1198, error in=w1213, "Strings[]"=w1210) -> (error out=w1226:errorcluster)  [unwired: 1 out]
      n474 = call "Certi Recall.vi"("큐 입력"=w1224, "NumRows"=w1191, "입력 클러스터"=w1190, "에러 입력"=w1226, "Func_ext in"=w1185) -> ("에러 출력"=w1225:errorcluster)  [unwired: 5 in, 1 out]
    }
    frame "Length_6_1", "Length_6_2" {
      n475 = call "Get Calproc.vi"("제목"=w1276, "에러 입력"=w1315, "Func_ext"=w1298) -> ("에러 출력"=w1314:errorcluster, "Condition"=w1269:string[][], "Func_ext Out"=w1310:string, "클러스터"=w1305:T7)  [unwired: 5 in]
      n476 = Unbundle By Name(w1306) -> ("Initialize 1.Measured"=w1260:refnum<vi>[], "Initialize 2.테이블"=w1289:refnum<vi>[], "Initialize 2.문자열"=w1266:refnum<vi>[], "Initialize 1.Condition"=w1299:refnum<vi>[], "Initialize 1.Spec"=w1308:refnum<vi>[])
      n477 = Unbundle By Name(w1305) -> ("Spec"=w1279:string[][], "CMC"=w1307:string[][], "NumRows"=w1280:u32)
      n478 = call "Variables Data IO.vi"("Select"=Cmd_Var_Data_IO."Condition", "error in"=w1314, "Data In"=w1269, "Func_ext"=w1310) -> ("error out"=w1302:errorcluster, "Func_ext Out"=w1301:string)  [unwired: 5 in, 1 out]
      n479 = call "Variables Data IO.vi"("Select"=Cmd_Var_Data_IO."Condition Default", "error in"=w1302, "Data In"=w1269, "Func_ext"=w1301) -> ("error out"=w1287:errorcluster, "Func_ext Out"=w1285:string)  [unwired: 5 in, 1 out]
      n480 = Index Array(array=w1308) -> (element=w1295:refnum<vi>)  [unwired: 1 in]
      n481 = call "STD Cal Data.vi"("error in"=w1287, "Func_ext"=w1285) -> ("error out"=w1286:errorcluster, "Data Out"=w1278:string[][], "Func_ext Out"=w1277:string)  [unwired: 5 in, 2 out]
      n482 = call "Get Spec.vi"("NumRows"=w1280, "Spec in"=w1279, "Spec Ref."=w1295, "error in"=w1286, "Condition in"=w1269, "Resolution in"=w1278, "Func_ext"=w1277) -> ("error out"=w1312:errorcluster, "Data Out"=w1309:string[][], "Spec Out"=w1296:string[][], "Func_ext Out"=w1311:string)  [unwired: 1 out]
      n483 = call "Match_CMC.vi"("CMC IN"=w1307, "error in"=w1312, "Condition IN"=w1309, "Func_ext"=w1311) -> ("error out"=w1297:errorcluster, "Func_ext out"=w1288:string)  [unwired: 4 in, 2 out]
      n484 = Index Array(array=w1299) -> (element=w1264:refnum<vi>)  [unwired: 1 in]
      n485 = call-poly "Cell Spacing.vi"("error in"=w1297, "Data in"=w1296, "테이블 참조 in"=w1295) -> ("error out"=w1294:errorcluster, "테이블 참조 Out"=w1293:refnum<vi>)  [unwired: 6 in, 1 out]
      n486 = property class="Tbl"(reference=w1293, error in=w1294, "Number of Columns"=u32 3 ("열의 개수")) -> (error out=w1291:errorcluster)  [unwired: 1 out]
      n487 = call-poly "Cell Spacing.vi"("error in"=w1291, "Data in"=w1269, "테이블 참조 in"=w1264) -> ("error out"=w1270:errorcluster, "열(U32)"=w1271:u32, "테이블 참조 Out"=w1290:refnum<vi>)  [unwired: 6 in]
      n488 = Index Array(array=w1278, index (col)=0 ("비활성화된 인덱스 (열)")) -> (element=w1273:string[])  [unwired: 1 in]
      n489 = call-poly "Table Initialize.vi"("행의 개수"=w1280, "Table Ref"=w1290, "Value"=w1269, "에러 입력"=w1270, "열의 개수"=w1271) -> ("에러 출력"=w1263:errorcluster)  [unwired: 4 in, 2 out]
      n490 = for {
        tunnel: w1273 -> [w1318] mode=indexing
        tunnel: [w1318] -> w1272 mode=indexing if=w1316
        n491 = call <vilib>:"Trim Whitespace.vi"("string"=w1318) -> ("trimmed string"=w1319:string)  [unwired: 1 in]
        n492 = Empty String/Path?(string/path=w1319) -> (empty?=w1317:bool)
        n493 = Not(x=w1317) -> (.not. x?=w1316:bool)
      }
      n494 = call "Extract String.vi"("Condition"=w1269) -> ("배열 2"=w1268:string[])  [unwired: 8 in, 2 out]
      n495 = call-poly "String Contents.vi"("문자 배열"=w1268, "참조 배열"=w1266, "에러 입력"=w1263) -> ("에러 출력"=w1267:errorcluster)  [unwired: 7 in, 1 out]
      n496 = Index Array(array=w1289) -> (element=w1283:refnum<vi>)  [unwired: 1 in]
      n497 = case shown="기본" w1275 {
        tunnel: [u32 4 ("열의 개수") u32 3 ("열의 개수")] -> w1274
        frame Default {
        }
        frame "10404-0" {
        }
      }
      n498 = Not A Number/Path/Refnum?(number/path/refnum=w1283) -> (NaN/Path/Refnum?=w1282:bool)
      n499 = case shown="거짓" w1282 {
        tunnel: w1267 -> [w1329 w1330]
        tunnel: [w1328 w1330] -> w1262
        tunnel: w1283 -> [w1327 _]
        tunnel: w1272 -> [w1326 _]
        tunnel: w1274 -> [w1322 _]
        frame False {
          n500 = Array Size(array=w1326) -> (size(s)=w1325:i32)
          n501 = Increment(x=w1325) -> (x+1=w1324:i32)
          n502 = property class="Tbl (엄격한)"(reference=w1327, error in=w1329, "Row Headers[]"=w1326, "Number of Rows"=w1324, "Value"=string[][] [] ("값"), "Number of Columns"=w1322) -> (error out=w1328:errorcluster)  [unwired: 1 out]
        }
        frame True {
        }
      }
      n503 = Build Array (concatenate)(w1264, w1295, w1260, w1289) -> (w1265:refnum<vi>[])
      n504 = call "Tbl Comp.vi"("배열"=w1265, "방향"=enum16{"수직", "수평"}."수평", "에러 입력"=w1262) -> ("에러 출력"=w1261:errorcluster)  [unwired: 6 in, 2 out]
      n505 = call "Certi Recall.vi"("큐 입력"=w1304, "NumRows"=w1280, "입력 클러스터"=w1303, "에러 입력"=w1261, "Func_ext in"=w1288) -> ("에러 출력"=w1259:errorcluster)  [unwired: 5 in, 1 out]
    }
    frame "Length_7" {
      n506 = call "Get Calproc.vi"("제목"=w1378, "에러 입력"=w1394, "Func_ext"=w1381) -> ("에러 출력"=w1393:errorcluster, "Condition"=w1347:string[][], "Func_ext Out"=w1389:string, "클러스터"=w1385:T7)  [unwired: 5 in]
      n507 = Unbundle By Name(w1386) -> ("Initialize 2.문자열"=w1355:refnum<vi>[], "Initialize 1.Condition"=w1339:refnum<vi>[], "Initialize 1.Spec"=w1337:refnum<vi>[], "Initialize 1.Measured"=w1336:refnum<vi>[], "Initialize 2.콤보박스"=w1367:refnum<vi>[])
      n508 = Unbundle By Name(w1385) -> ("Data"=w1345:string[][], "Spec"=w1379:string[][], "CMC"=w1387:string[][], "NumRows"=w1331:u32)
      n509 = case shown="\"10232-2\"" w1346 {
        tunnel: [w1397 w1413] -> w1372
        tunnel: [w1396 w1412] -> w1371
        tunnel: w1347 -> [w1395 w1409]
        tunnel: [w1395 w1406] -> w1344
        tunnel: w1345 -> [_ w1411]
        frame Default {
          n510 = for {
            tunnel: w1395 -> [w1402] mode=indexing
            tunnel: [w1403] -> w1397 mode=indexing
            tunnel: [w1398] -> w1396 mode=indexing
            n511 = Index Array(array=w1402) -> (element #1=w1401:string, element #2=w1400:string)  [unwired: 2 in]
            n512 = Format Into String(format string="%s %s" ("포맷 문자열"), w1401, w1400) -> (resulting string=w1398:string)  [unwired: 2 in, 1 out]
            n513 = Build Array("0" ("원소"), "μm" ("원소")) -> (w1403:string[])
          }
        }
        frame "10232-2" {
          n514 = for {
            tunnel: w1409 -> [w1418] mode=indexing
            tunnel: [w1419] -> w1413 mode=indexing
            tunnel: [w1414] -> w1412 mode=indexing
            n515 = Index Array(array=w1418) -> (element #1=w1417:string, element #2=w1416:string)  [unwired: 2 in]
            n516 = Format Into String(format string="%s %s" ("포맷 문자열"), w1417, w1416) -> (resulting string=w1414:string)  [unwired: 2 in, 1 out]
            n517 = Build Array("0" ("원소"), "μm" ("원소")) -> (w1419:string[])
          }
          n518 = Index Array(array=w1411, index (col)=8 ("비활성화된 인덱스 (열)")) -> (element=w1408:string[])  [unwired: 1 in]
          n519 = Insert Into Array(array=w1409, index (col)=0 ("비활성화된 인덱스 (열)"), new element=w1408) -> (w1406:string[][])  [unwired: 1 in]
        }
      }
      n520 = Index Array(array=w1367) -> (element=w1359:refnum<vi>)  [unwired: 1 in]
      n521 = Index Array(array=w1337) -> (element=w1380:refnum<vi>)  [unwired: 1 in]
      n522 = call "Variables Data IO.vi"("Select"=Cmd_Var_Data_IO."Condition", "error in"=w1393, "Data In"=w1344, "Func_ext"=w1389) -> ("error out"=w1351:errorcluster, "Func_ext Out"=w1373:string)  [unwired: 5 in, 1 out]
      n523 = call "Variables Data IO.vi"("Select"=Cmd_Var_Data_IO."Condition Default", "error in"=w1351, "Data In"=w1372, "Func_ext"=w1373) -> ("error out"=w1369:errorcluster, "Func_ext Out"=w1358:string)  [unwired: 5 in, 1 out]
      n524 = call "Select E_M Range.vi"("Data"=w1344, "STD Select Ref."=w1359, "에러 입력"=w1369, "Func in"=w1358) -> ("에러 출력"=w1368:errorcluster, "STD Select Value"=w1370:string, "Func out"=w1357:string, "STD Resolution"=w1360:string[][])  [unwired: 4 in]
      n525 = Array Size(array=w1344) -> (size(s)=w1343:i32[])
      n526 = call "STD Cal Data.vi"("error in"=w1368, "문자열"=w1370, "Func_ext"=w1357) -> ("error out"=w1366:errorcluster, "Data Out"=w1376:string[][], "Func_ext Out"=w1364:string, "Data Out 2"=w1361:string[])  [unwired: 4 in, 1 out]
      n527 = Index Array(array=w1343) -> (element #2=w1342:i32)  [unwired: 2 in, 1 out]
      n528 = call "Variables Data IO.vi"("Select"=Cmd_Var_Data_IO."Resolution", "error in"=w1366, "Data In"=w1360, "Func_ext"=w1364) -> ("error out"=w1365:errorcluster, "Func_ext Out"=w1363:string)  [unwired: 5 in, 1 out]
      n529 = call "Get Spec.vi"("NumRows"=w1331, "Spec in"=w1379, "Spec Ref."=w1380, "error in"=w1365, "Condition in"=w1344, "Resolution in"=w1360, "Func_ext"=w1363) -> ("error out"=w1391:errorcluster, "Data Out"=w1388:string[][], "Func_ext Out"=w1390:string)  [unwired: 2 out]
      n530 = call "Match_CMC.vi"("CMC IN"=w1387, "error in"=w1391, "Condition IN"=w1388, "Func_ext"=w1390) -> ("error out"=w1352:errorcluster, "Func_ext out"=w1349:string)  [unwired: 4 in, 2 out]
      n531 = Index Array(array=w1339) -> (element #1=w1338:refnum<vi>, element #2=w1377:refnum<vi>)  [unwired: 2 in]
      n532 = call-poly "Table Initialize.vi"("행의 개수"=w1331, "Table Ref"=w1338, "Value"=w1344, "에러 입력"=w1352, "열의 개수"=w1342) -> ("에러 출력"=w1354:errorcluster, "Bottom"=w1374:i32)  [unwired: 4 in, 1 out]
      n533 = call-poly "Cell Spacing.vi"("Row Header in"=w1371, "Col Header in"=w1361, "error in"=w1354, "Data in"=w1376, "테이블 참조 in"=w1377) -> ("error out"=w1353:errorcluster, "테이블 참조 Out"=w1375:refnum<vi>)  [unwired: 4 in, 1 out]
      n534 = Build Array (concatenate)(w1338, w1337, w1336) -> (w1335:refnum<vi>[])
      n535 = property on="STD set" class="Tbl"(reference=w1375, error in=w1353, "Top"=w1374, "Number of Rows"=w1331) -> (error out=w1334:errorcluster)  [unwired: 1 out]
      n536 = call "Meas2 status_1D Arr.vi"("행의 개수"=w1331, "입력 클러스터"=w1350, "에러 입력"=w1334, "Func_ext"=w1349) -> ("에러 출력"=w1333:errorcluster, "Func_ext Out"=w1348:string)  [unwired: 6 in]
      n537 = call "Tbl Comp.vi"("배열"=w1335, "방향"=enum16{"수직", "수평"}."수평", "에러 입력"=w1333) -> ("에러 출력"=w1341:errorcluster)  [unwired: 6 in, 2 out]
      n538 = call "Extract String.vi"("Condition"=w1344) -> ("배열 2"=w1356:string[])  [unwired: 8 in, 2 out]
      n539 = call-poly "String Contents.vi"("문자 배열"=w1356, "참조 배열"=w1355, "에러 입력"=w1341) -> ("에러 출력"=w1332:errorcluster)  [unwired: 7 in, 1 out]
      n540 = call "Certi Recall.vi"("큐 입력"=w1383, "NumRows"=w1331, "입력 클러스터"=w1350, "에러 입력"=w1332, "Func_ext in"=w1348) -> ("에러 출력"=w1384:errorcluster)  [unwired: 5 in, 1 out]
    }
    frame "Length_8" {
      n541 = Unbundle By Name(w1476) -> ("Initialize 2.콤보박스"=w1440:refnum<vi>[], "Initialize 2.문자열"=w1443:refnum<vi>[], "Initialize 1.Resolution"=w1478:refnum<vi>[], "Initialize 1.Spec"=w1464:refnum<vi>[], "Initialize 1.Condition"=w1488:refnum<vi>[], "Initialize 2.콤보박스"=w1468:refnum<vi>[])
      n542 = call "Get Calproc.vi"("제목"=w1451, "에러 입력"=w1489, "Func_ext"=w1480) -> ("에러 출력"=w1487:errorcluster, "Condition"=w1445:string[][], "Func_ext Out"=w1481:string, "클러스터"=w1472:T7)  [unwired: 5 in]
      n543 = Unbundle By Name(w1472) -> ("Data"=w1459:string[][], "Spec"=w1455:string[][], "CMC"=w1463:string[][], "Resolution"=w1438:string[][], "NumRows"=w1452:u32, "Condition"=w1426:string[][])
      n544 = call "Variables Data IO.vi"("Select"=Cmd_Var_Data_IO."Condition", "error in"=w1487, "Data In"=w1445, "Func_ext"=w1481) -> ("error out"=w1473:errorcluster, "Func_ext Out"=w1483:string)  [unwired: 5 in, 1 out]
      n545 = call "Variables Data IO.vi"("Select"=Cmd_Var_Data_IO."Condition Default", "error in"=w1473, "Data In"=w1445, "Func_ext"=w1483) -> ("error out"=w1432:errorcluster, "Func_ext Out"=w1448:string)  [unwired: 5 in, 1 out]
      n546 = Index Array(array=w1468, index=2 ("인덱스")) -> (element=w1449:refnum<vi>)
      n547 = call "Select E_M Range.vi"("Data"=w1459, "STD Select Ref."=w1449, "에러 입력"=w1432, "Func in"=w1448) -> ("에러 출력"=w1466:errorcluster, "STD Select Value"=w1460:string, "Func out"=w1447:string, "STD Resolution"=w1454:string[][])  [unwired: 4 in]
      n548 = call "STD Cal Data.vi"("error in"=w1466, "Data in"=w1459, "문자열"=w1460, "Func_ext"=w1447) -> ("error out"=w1433:errorcluster, "Data Out"=w1456:string[][], "Func_ext Out"=w1429:string, "Data Out 2"=w1457:string[])  [unwired: 3 in, 1 out]
      n549 = Index Array(array=w1488) -> (element #1=w1475:refnum<vi>, element #2=w1431:refnum<vi>)  [unwired: 2 in]
      n550 = call-poly "Table Initialize.vi"("행의 개수"=w1452, "Table Ref"=w1475, "Value"=w1445, "에러 입력"=w1433) -> ("에러 출력"=w1467:errorcluster, "Bottom"=w1477:i32)  [unwired: 5 in, 1 out]
      n551 = for {
        tunnel: w1445 -> [w1494] mode=indexing
        tunnel: [w1490] -> w1450 mode=indexing
        n552 = Index Array(array=w1494) -> (element #1=w1493:string, element #2=w1492:string)  [unwired: 2 in]
        n553 = Format Into String(format string="%s %s" ("포맷 문자열"), w1493, w1492) -> (resulting string=w1490:string)  [unwired: 2 in, 1 out]
      }
      n554 = property class="Tbl (엄격한)"(reference=w1431, error in=w1467, "Top"=w1477, "Number of Rows"=w1452) -> (reference out=w1469:refnum<vi>, error out=w1458:errorcluster)
      n555 = Index Array(array=w1464) -> (element=w1474:refnum<vi>)  [unwired: 1 in]
      n556 = call-poly "Cell Spacing.vi"("Row Header in"=w1450, "Col Header in"=w1457, "error in"=w1458, "Data in"=w1456, "테이블 참조 in"=w1469) -> ("error out"=w1430:errorcluster)  [unwired: 4 in, 2 out]
      n557 = Index Array(array=w1478) -> (element=w1453:refnum<vi>)  [unwired: 1 in]
      n558 = call "Variables Data IO.vi"("Select"=Cmd_Var_Data_IO."Resolution Default", "error in"=w1430, "Data In"=w1454, "Func_ext"=w1429) -> ("error out"=w1428:errorcluster, "Func_ext Out"=w1427:string)  [unwired: 5 in, 1 out]
      n559 = call "Get Spec.vi"("NumRows"=w1452, "Spec in"=w1455, "Spec Ref."=w1474, "error in"=w1428, "Condition in"=w1445, "Resolution in"=w1454, "Func_ext"=w1427) -> ("error out"=w1484:errorcluster, "Data Out"=w1479:string[][], "Func_ext Out"=w1482:string)  [unwired: 2 out]
      n560 = call "Match_CMC.vi"("CMC IN"=w1463, "error in"=w1484, "Condition IN"=w1479, "Func_ext"=w1482) -> ("error out"=w1465:errorcluster, "Func_ext out"=w1462:string)  [unwired: 4 in, 2 out]
      n561 = call "Create Resolution.vi"("행의 개수"=w1452, "Table Ref"=w1453, "에러 입력(에러 없음)"=w1465, "Resolution"=w1438, "Func_ext"=w1462) -> ("에러 출력"=w1442:errorcluster, "Func_ext 출력"=w1425:string)  [unwired: 4 in, 1 out]
      n562 = call "Extract String.vi"("Resolution"=w1438, "Condition"=w1426) -> ("배열 1"=w1439:string[], "배열 2"=w1444:string[])  [unwired: 7 in, 1 out]
      n563 = call-poly "String Contents.vi"("문자 배열"=w1444, "참조 배열"=w1443, "에러 입력"=w1442) -> ("에러 출력"=w1441:errorcluster)  [unwired: 7 in, 1 out]
      n564 = call-poly "String Contents.vi"("문자 배열"=w1439, "참조 배열"=w1440, "에러 입력"=w1441) -> ("에러 출력"=w1435:errorcluster, "참조"=w1436:refnum<vi>)  [unwired: 7 in]
      n565 = property on="표시형식" class="CmbBox"(reference=w1436, error in=w1435, "Strings[]"=w1437) -> (error out=w1424:errorcluster)  [unwired: 1 out]
      n566 = call "Meas2 status_1D Arr.vi"("입력 클러스터"=w1446, "에러 입력"=w1424, "Func_ext"=w1425) -> ("에러 출력"=w1422:errorcluster, "Func_ext Out"=w1423:string)  [unwired: 7 in]
      n567 = call "Certi Recall.vi"("큐 입력"=w1470, "NumRows"=w1452, "입력 클러스터"=w1446, "에러 입력"=w1422, "Func_ext in"=w1423) -> ("에러 출력"=w1471:errorcluster)  [unwired: 5 in, 1 out]
    }
    frame "Length_9" {
      w1496 = "mm" ("포맷 문자열")
      n568 = call "Get Calproc.vi"("제목"=w1506, "에러 입력"=w1567, "Func_ext"=w1565) -> ("에러 출력"=w1566:errorcluster, "Func_ext Out"=w1532:string, "클러스터"=w1563:T7)  [unwired: 5 in, 1 out]
      n569 = Unbundle By Name(w1564) -> ("Initialize 1.Spec"=w1548:refnum<vi>[], "Initialize 1.Condition"=w1562:refnum<vi>[], "Initialize 2.콤보박스"=w1536:refnum<vi>[], "Initialize 2.문자열"=w1500:refnum<vi>[])  [unwired: 1 out]
      n570 = Unbundle By Name(w1563) -> ("Temp_1"=w1559:string[][], "Spec"=w1510:string[][], "CMC"=w1546:string[][], "NumRows"=w1511:u32)
      n571 = for {
        tunnel: w1500 -> [w1571] mode=indexing
        tunnel: [w1570] -> w1503 mode=indexing
        shift-right: [w1569] -> _
        shift-left: _ -> [w1568]
        n572 = property class="Str"(reference=w1571, error in=w1568) -> (error out=w1569:errorcluster, "Value"=w1570:string)  [unwired: 1 out]
      }
      n573 = Index Array(array=w1536) -> (element=w1535:refnum<vi>)  [unwired: 1 in]
      n574 = Index Array(array=w1503) -> (element #1=w1499:string, element #2=w1502:string, element #3=w1501:string)  [unwired: 3 in]
      n575 = property on="단위" class="CmbBox"(reference=w1535, error in=w1566) -> (error out=w1498:errorcluster, "Value"=w1529:string)  [unwired: 1 out]
      n576 = Build Array(w1502, w1499, w1529, w1501) -> (w1557:string[])
      n577 = call "Unit Conversion.vi"("환산단위"=w1496, "입력단위"=w1529, "입력값"=w1502) -> ("환산값 (DBL)"=w1526:dbl, "환산값 (string)"=w1534:string)  [unwired: 3 in, 4 out]
      n578 = call "Unit Conversion.vi"("환산단위"=w1496, "입력단위"=w1529, "입력값"=w1499) -> ("환산값 (DBL)"=w1519:dbl, "환산값 (string)"=w1533:string)  [unwired: 3 in, 4 out]
      n579 = Fract/Exp String To Number(string=w1501) -> (number=w1518:dbl)  [unwired: 3 in, 1 out]
      n580 = Index Array(array=w1562) -> (element=w1561:refnum<vi>)  [unwired: 1 in]
      n581 = Build Array(w1557) -> (w1556:string[][])
      n582 = Add(x=w1526, y=w1519) -> (x+y=w1523:dbl)
      n583 = Index Array(array=w1548) -> (element #1=w1547:refnum<vi>, element #2=w1512:refnum<vi>)  [unwired: 2 in]
      n584 = Multiply(x=w1523, y=w1518) -> (x*y=w1541:dbl)
      n585 = Format Into String(format string="%#f" ("포맷 문자열"), w1541) -> (resulting string=w1539:string)  [unwired: 2 in, 1 out]
      n586 = call "Variables Data IO.vi"("Select"=Cmd_Var_Data_IO."Condition_Temp", "error in"=w1498, "Data In"=w1556, "Func_ext"=w1532) -> ("error out"=w1522:errorcluster, "Func_ext Out"=w1521:string)  [unwired: 5 in, 1 out]
      n587 = Build Array(w1533, w1533, w1534, w1534, w1534, w1534) -> (w1538:string[])
      n588 = Build Array(w1533, w1533, w1539, w1539, w1539, w1539) -> (w1542:string[])
      n589 = for {
        tunnel: w1542 -> [w1591] mode=indexing
        tunnel: "mm" ("포맷 문자열") -> [w1594]
        tunnel: [w1593] -> w1520 mode=indexing
        tunnel: w1538 -> [w1592] mode=indexing
        n590 = Build Array(w1591, w1592, w1594) -> (w1593:string[])
      }
      n591 = Insert Into Array(array=w1520, index (col)=0 ("비활성화된 인덱스 (열)"), new element=w1559) -> (w1505:string[][])  [unwired: 1 in]
      n592 = call "Variables Data IO.vi"("Select"=Cmd_Var_Data_IO."Condition", "error in"=w1522, "Data In"=w1505, "Func_ext"=w1521) -> ("error out"=w1551:errorcluster, "Func_ext Out"=w1550:string)  [unwired: 5 in, 1 out]
      n593 = call-poly "Table Initialize.vi"("행의 개수"=w1511, "Table Ref"=w1561, "Value"=w1505, "에러 입력"=w1551) -> ("에러 출력"=w1537:errorcluster)  [unwired: 5 in, 2 out]
      n594 = call "STD Cal Data.vi"("error in"=w1537, "Func_ext"=w1550) -> ("error out"=w1530:errorcluster, "Data Out"=w1509:string[][], "Func_ext Out"=w1531:string, "Cal STD"=w1524:string[][])  [unwired: 5 in, 1 out]
      n595 = Index Array(array=w1524, index (row)=0 ("인덱스 (행)"), index (col)=9 ("비활성화된 인덱스 (열)")) -> (element=w1497:string)
      n596 = for {
        tunnel: [w1589] -> w1525 mode=indexing
        tunnel: w1497 -> [w1587]
        tunnel: w1509 -> [_] mode=indexing
        n597 = Build Array("Digital", w1587, "mm" ("입력단위")) -> (w1589:string[])
      }
      n598 = call "Number Format.vi"("입력값"=w1497) -> ("정밀도(단위적용)"=w1516:i32)  [unwired: 10 in]
      n599 = call "Create Resolution.vi"("에러 입력(에러 없음)"=w1530, "Resolution"=w1525, "Func_ext"=w1531) -> ("에러 출력"=w1549:errorcluster, "Resolution Out"=w1508:string[][], "Func_ext 출력"=w1507:string)  [unwired: 6 in]
      n600 = call "Get Spec.vi"("NumRows"=w1511, "Spec in"=w1510, "Spec Ref."=w1547, "error in"=w1549, "Condition in"=w1509, "Resolution in"=w1508, "Func_ext"=w1507) -> ("error out"=w1515:errorcluster, "Data Out"=w1544:string[][], "Spec Out"=w1517:string[][], "Func_ext Out"=w1545:string)  [unwired: 1 out]
      n601 = for {
        tunnel: w1519 -> [w1586]
        tunnel: w1518 -> [w1584]
        tunnel: [w1575] -> w1504 mode=indexing
        tunnel: w1517 -> [w1574] mode=indexing
        tunnel: w1516 -> [w1580]
        i -> [w1578]
        w1572 = 2 ("인덱스")
        n602 = Fract/Exp String To Number(string=w1574) -> (number=w1573:dbl[])  [unwired: 3 in, 1 out]
        n603 = Index Array(array=w1574, index=w1572) -> (element=w1581:string)
        n604 = Add(x=w1573, y=w1586) -> (x+y=w1585:dbl[])
        n605 = Greater?(x=w1578, y=1) -> (0:w1576:bool)
        n606 = Multiply(x=w1585, y=w1584) -> (x*y=w1583:dbl[])
        n607 = Number To Fractional String(number=w1583, precision (6)=w1580) -> (F-format string=w1582:string[])  [unwired: 2 in]
        n608 = Replace Array Subset(array=w1582, new element=w1581, index=w1572) -> (w1579:string[])
        n609 = Select(t=w1579, s=w1576, f=w1574) -> (s? t:f=w1575:string[])
      }
      n610 = call "Match_CMC.vi"("CMC IN"=w1546, "error in"=w1515, "Condition IN"=w1544, "Func_ext"=w1545) -> ("error out"=w1514:errorcluster, "Func_ext out"=w1543:string)  [unwired: 4 in, 2 out]
      n611 = call-poly "Table Initialize.vi"("행의 개수"=w1511, "Table Ref"=w1512, "Value"=w1504, "에러 입력"=w1514) -> ("에러 출력"=w1513:errorcluster)  [unwired: 5 in, 2 out]
      n612 = call "Certi Recall.vi"("큐 입력"=w1554, "입력 클러스터"=w1553, "에러 입력"=w1513, "Func_ext in"=w1543) -> ("에러 출력"=w1552:errorcluster)  [unwired: 6 in, 1 out]
    }
    frame "Magnification_1" {
      n613 = Unbundle By Name(w1641) -> ("Initialize 2.문자열"=w1617:refnum<vi>[], "Initialize 1.Condition"=w1631:refnum<vi>[], "Initialize 1.Spec"=w1643:refnum<vi>[], "Initialize 1.Resolution"=w1632:refnum<vi>[], "Initialize 2.테이블"=w1621:refnum<vi>[])
      n614 = call "Get Calproc.vi"("제목"=w1625, "에러 입력"=w1649, "Func_ext"=w1645) -> ("에러 출력"=w1599:errorcluster, "Condition"=w1597:string[][], "Func_ext Out"=w1601:string, "클러스터"=w1637:T7)  [unwired: 5 in]
      n615 = Unbundle By Name(w1637) -> ("Spec"=w1630:string[][], "CMC"=w1642:string[][], "NumRows"=w1604:u32)
      n616 = Index Array(array=w1621) -> (element=w1615:refnum<vi>)  [unwired: 1 in]
      n617 = call "Variables Data IO.vi"("Select"=Cmd_Var_Data_IO."Condition Default", "error in"=w1599, "Data In"=w1597, "Func_ext"=w1601) -> ("error out"=w1598:errorcluster, "Func_ext Out"=w1600:string)  [unwired: 5 in, 1 out]
      n618 = property class="Tbl (엄격한)"(reference=w1615, error in=w1598, "Number of Rows"=w1604) -> (error out=w1614:errorcluster, "Value"=w1613:string[][])  [unwired: 1 out]
      n619 = Index Array(array=w1613, index (col)=0 ("비활성화된 인덱스 (열)")) -> (element=w1609:string[])  [unwired: 1 in]
      n620 = Fract/Exp String To Number(string=w1609) -> (number=w1611:dbl[])  [unwired: 3 in, 1 out]
      n621 = call "Extract String.vi"("Condition"=w1597) -> ("배열 2"=w1596:string[], "측정범위"=w1595:dbl[])  [unwired: 8 in, 1 out]
      n622 = Multiply(x=w1611, y=w1595) -> (x*y=w1610:dbl[])
      n623 = for {
        tunnel: w1597 -> [w1662] mode=indexing
        tunnel: "mm" ("포맷 문자열") -> [w1654]
        tunnel: [w1659] -> w1605 mode=indexing
        tunnel: w1610 -> [w1656] mode=indexing
        tunnel: w1609 -> [w1655] mode=indexing
        n624 = Format Into String(format string="%#f" ("포맷 문자열"), w1656) -> (resulting string=w1657:string)  [unwired: 2 in, 1 out]
        n625 = Index Array(array=w1662) -> (element #1=w1661:string, element #2=w1660:string)  [unwired: 2 in]
        n626 = Build Array(w1655, w1654, w1661, w1660, w1657, w1654) -> (w1659:string[])
      }
      n627 = call "Variables Data IO.vi"("Select"=Cmd_Var_Data_IO."Condition", "error in"=w1614, "Data In"=w1605, "Func_ext"=w1600) -> ("error out"=w1603:errorcluster, "Func_ext Out"=w1602:string)  [unwired: 5 in, 1 out]
      n628 = Index Array(array=w1632) -> (element=w1629:refnum<vi>)  [unwired: 1 in]
      n629 = call "STD Cal Data.vi"("error in"=w1603, "Func_ext"=w1602) -> ("error out"=w1620:errorcluster, "Func_ext Out"=w1616:string, "Data Out 2"=w1608:string[])  [unwired: 5 in, 2 out]
      n630 = Index Array(array=w1643) -> (element=w1639:refnum<vi>)  [unwired: 1 in]
      n631 = Index Array(array=w1608) -> (element=w1607:string)  [unwired: 1 in]
      n632 = Index Array(array=w1631) -> (element=w1640:refnum<vi>)  [unwired: 1 in]
      n633 = Build Array (concatenate)(w1596, w1607) -> (w1624:string[])
      n634 = for {
        tunnel: w1607 -> [w1653]
        tunnel: [w1650] -> w1606 mode=indexing
        tunnel: w1605 -> [_] mode=indexing
        n635 = Build Array("Analog" ("원소"), w1653, "mm" ("원소")) -> (w1650:string[])
      }
      n636 = call "Create Resolution.vi"("행의 개수"=w1604, "Table Ref"=w1629, "에러 입력(에러 없음)"=w1620, "Resolution"=w1606, "Func_ext"=w1616) -> ("에러 출력"=w1627:errorcluster, "Resolution Out"=w1628:string[][], "Func_ext 출력"=w1626:string)  [unwired: 4 in]
      n637 = call "Get Spec.vi"("NumRows"=w1604, "Spec in"=w1630, "Spec Ref."=w1639, "error in"=w1627, "Condition in"=w1605, "Resolution in"=w1628, "Func_ext"=w1626) -> ("error out"=w1647:errorcluster, "Data Out"=w1644:string[][], "Func_ext Out"=w1646:string)  [unwired: 2 out]
      n638 = call "Match_CMC.vi"("CMC IN"=w1642, "error in"=w1647, "Condition IN"=w1644, "Func_ext"=w1646) -> ("error out"=w1638:errorcluster, "Func_ext out"=w1623:string)  [unwired: 4 in, 2 out]
      n639 = call-poly "Table Initialize.vi"("행의 개수"=w1604, "Table Ref"=w1640, "Value"=w1605, "에러 입력"=w1638) -> ("에러 출력"=w1619:errorcluster)  [unwired: 5 in, 2 out]
      n640 = call-poly "String Contents.vi"("문자 배열"=w1624, "참조 배열"=w1617, "에러 입력"=w1619) -> ("에러 출력"=w1618:errorcluster)  [unwired: 7 in, 1 out]
      n641 = call "Certi Recall.vi"("큐 입력"=w1635, "NumRows"=w1604, "입력 클러스터"=w1634, "에러 입력"=w1618, "Func_ext in"=w1623) -> ("에러 출력"=w1636:errorcluster)  [unwired: 5 in, 1 out]
    }
    frame "Squareness_1" {
      n642 = Unbundle By Name(w1689) -> ("Initialize 2.콤보박스"=w1667:refnum<vi>[], "Initialize 2.문자열"=w1680:refnum<vi>[], "Initialize 1.Condition"=w1681:refnum<vi>[], "Initialize 1.Spec"=w1699:refnum<vi>[], "Initialize 1.Resolution"=w1698:refnum<vi>[])
      n643 = call "Get Calproc.vi"("제목"=w1688, "에러 입력"=w1686, "Func_ext"=w1687) -> ("에러 출력"=w1716:errorcluster, "Condition"=w1712:string[][], "Func_ext Out"=w1714:string, "클러스터"=w1707:T7)  [unwired: 5 in]
      n644 = Unbundle By Name(w1707) -> ("Temp_1"=w1713:string[][], "Resolution"=w1704:string[][], "Spec"=w1708:string[][], "CMC"=w1700:string[][], "Data"=w1663:string[][], "NumRows"=w1684:u32, "Temp_1"=w1678:string[][], "Condition"=w1673:string[][], "Resolution"=w1671:string[][])
      n645 = call "Array Size.vi"("Data in"=w1678) -> ("열(U32)"=w1668:u32)  [unwired: 7 in, 3 out]
      n646 = call "Extract String.vi"("Resolution"=w1671, "Condition"=w1673) -> ("배열 1"=w1674:string[], "배열 2"=w1672:string[])  [unwired: 7 in, 1 out]
      n647 = call "Variables Data IO.vi"("Select"=Cmd_Var_Data_IO."Condition_Temp", "error in"=w1716, "Data In"=w1713, "Func_ext"=w1714) -> ("error out"=w1717:errorcluster, "Func_ext Out"=w1715:string)  [unwired: 5 in, 1 out]
      n648 = Index Array(array=w1698) -> (element=w1711:refnum<vi>)  [unwired: 1 in]
      n649 = call "Variables Data IO.vi"("Select"=Cmd_Var_Data_IO."Condition", "error in"=w1717, "Data In"=w1663, "Func_ext"=w1715) -> ("error out"=w1705:errorcluster, "Func_ext Out"=w1695:string)  [unwired: 5 in, 1 out]
      n650 = Index Array(array=w1699) -> (element=w1703:refnum<vi>)  [unwired: 1 in]
      n651 = call "Variables Data IO.vi"("Select"=Cmd_Var_Data_IO."Condition Default", "error in"=w1705, "Data In"=w1712, "Func_ext"=w1695) -> ("error out"=w1718:errorcluster, "Func_ext Out"=w1719:string)  [unwired: 5 in, 1 out]
      n652 = Index Array(array=w1681) -> (element #1=w1701:refnum<vi>)  [unwired: 2 in, 1 out]
      n653 = call "Create Resolution.vi"("행의 개수"=w1684, "Table Ref"=w1711, "에러 입력(에러 없음)"=w1718, "Resolution"=w1704, "Func_ext"=w1719) -> ("에러 출력"=w1694:errorcluster, "Resolution Out"=w1709:string[][], "Func_ext 출력"=w1710:string)  [unwired: 4 in]
      n654 = Add(x=u32 2 ("y"), y=w1668) -> (x+y=w1720:u32)
      n655 = call "Get Spec.vi"("NumRows"=w1684, "Spec in"=w1708, "Spec Ref."=w1703, "error in"=w1694, "Condition in"=w1663, "Resolution in"=w1709, "Func_ext"=w1710) -> ("error out"=w1693:errorcluster, "Data Out"=w1697:string[][], "Func_ext Out"=w1696:string)  [unwired: 2 out]
      n656 = call "Match_CMC.vi"("CMC IN"=w1700, "error in"=w1693, "Condition IN"=w1697, "Func_ext"=w1696) -> ("error out"=w1666:errorcluster, "Func_ext out"=w1679:string)  [unwired: 4 in, 2 out]
      n657 = call "STD Cal Data.vi"("error in"=w1666, "Func_ext"=w1679) -> ("error out"=w1665:errorcluster, "Func_ext Out"=w1682:string)  [unwired: 5 in, 3 out]
      n658 = call-poly "Table Initialize.vi"("행의 개수"=w1684, "Table Ref"=w1701, "Value"=w1663, "에러 입력"=w1665, "열의 개수"=w1720) -> ("에러 출력"=w1664:errorcluster)  [unwired: 4 in, 2 out]
      n659 = call-poly "String Contents.vi"("문자 배열"=w1672, "참조 배열"=w1680, "에러 입력"=w1664) -> ("에러 출력"=w1670:errorcluster)  [unwired: 7 in, 1 out]
      n660 = call-poly "String Contents.vi"("문자 배열"=w1674, "참조 배열"=w1667, "에러 입력"=w1670) -> ("에러 출력"=w1676:errorcluster, "참조"=w1675:refnum<vi>)  [unwired: 7 in]
      n661 = property on="표시형식" class="CmbBox"(reference=w1675, error in=w1676, "Strings[]"=w1677) -> (error out=w1669:errorcluster)  [unwired: 1 out]
      n662 = call "Certi Recall.vi"("큐 입력"=w1690, "NumRows"=w1684, "입력 클러스터"=w1683, "에러 입력"=w1669, "Func_ext in"=w1682) -> ("에러 출력"=w1685:errorcluster)  [unwired: 5 in, 1 out]
    }
    frame "Squareness_2" {
      n663 = call "Get Calproc.vi"("제목"=w1758, "에러 입력"=w1756, "Func_ext"=w1757) -> ("에러 출력"=w1777:errorcluster, "Condition"=w1721:string[][], "Func_ext Out"=w1776:string, "클러스터"=w1772:T7)  [unwired: 5 in]
      n664 = Unbundle By Name(w1759) -> ("Initialize 2.문자열"=w1752:refnum<vi>[], "Initialize 1.Spec"=w1745:refnum<vi>[], "Initialize 2.콤보박스"=w1739:refnum<vi>[], "Initialize 1.Condition"=w1744:refnum<vi>[])
      n665 = Unbundle By Name(w1772) -> ("Data"=w1726:string[][], "Spec"=w1773:string[][], "CMC"=w1768:string[][], "NumRows"=w1754:u32)
      n666 = call "Variables Data IO.vi"("Select"=Cmd_Var_Data_IO."Condition Default", "error in"=w1777, "Data In"=w1721, "Func_ext"=w1776) -> ("error out"=w1771:errorcluster, "Func_ext Out"=w1765:string)  [unwired: 5 in, 1 out]
      n667 = Index Array(array=w1726, index (col)=7 ("비활성화된 인덱스 (열)")) -> (element=w1724:string[])  [unwired: 1 in]
      n668 = Insert Into Array(array=w1721, index (col)=0 ("비활성화된 인덱스 (열)"), new element=w1724) -> (w1722:string[][])  [unwired: 1 in]
      n669 = Index Array(array=w1744) -> (element=w1769:refnum<vi>)  [unwired: 1 in]
      n670 = call "Variables Data IO.vi"("Select"=Cmd_Var_Data_IO."Condition", "error in"=w1771, "Data In"=w1722, "Func_ext"=w1765) -> ("error out"=w1747:errorcluster, "Func_ext Out"=w1743:string)  [unwired: 5 in, 1 out]
      n671 = Index Array(array=w1739) -> (element=w1749:refnum<vi>)  [unwired: 1 in]
      n672 = call-poly "Table Initialize.vi"("행의 개수"=w1754, "Table Ref"=w1769, "Value"=w1722, "에러 입력"=w1747) -> ("에러 출력"=w1746:errorcluster)  [unwired: 5 in, 2 out]
      n673 = call "Select E_M Range.vi"("STD Select Ref."=w1749, "에러 입력"=w1746, "Func in"=w1743) -> ("에러 출력"=w1751:errorcluster, "STD Select Value"=w1750:string, "Func out"=w1742:string)  [unwired: 5 in, 1 out]
      n674 = call "STD Cal Data.vi"("error in"=w1751, "문자열"=w1750, "Func_ext"=w1742) -> ("error out"=w1738:errorcluster, "Data Out"=w1737:string[][], "Func_ext Out"=w1741:string)  [unwired: 4 in, 2 out]
      n675 = Index Array(array=w1737, index (row)=0 ("인덱스 (행)"), index (col)=24 ("비활성화된 인덱스 (열)")) -> (element=w1733:string)
      n676 = for {
        tunnel: w1721 -> [w1783] mode=indexing
        tunnel: [w1782] -> w1734 mode=indexing
        tunnel: w1733 -> [w1787]
        tunnel: [w1784] -> w1731 mode=indexing
        tunnel: w1726 -> [w1781] mode=indexing
        n677 = Index Array(array=w1781, index #1=5 ("인덱스")) -> (element #1=w1779:string, element #2=w1778:string)  [unwired: 1 in]
        n678 = Build Array("Digital" ("원소"), w1787, "μm" ("원소")) -> (w1784:string[])
        n679 = Build Array (concatenate)(w1783, w1779, w1778) -> (w1782:string[])
      }
      n680 = Index Array(array=w1745) -> (element=w1770:refnum<vi>)  [unwired: 1 in]
      n681 = call "Create Resolution.vi"("행의 개수"=w1754, "에러 입력(에러 없음)"=w1738, "Resolution"=w1731, "Func_ext"=w1741) -> ("에러 출력"=w1764:errorcluster, "Resolution Out"=w1774:string[][], "Func_ext 출력"=w1775:string)  [unwired: 5 in]
      n682 = call "Get Spec.vi"("NumRows"=w1754, "Spec in"=w1773, "Spec Ref."=w1770, "error in"=w1764, "Condition in"=w1734, "Resolution in"=w1774, "Func_ext"=w1775) -> ("error out"=w1763:errorcluster, "Data Out"=w1767:string[][], "Func_ext Out"=w1766:string)  [unwired: 2 out]
      n683 = call "Match_CMC.vi"("CMC IN"=w1768, "error in"=w1763, "Condition IN"=w1767, "Func_ext"=w1766) -> ("error out"=w1732:errorcluster, "Func_ext out"=w1740:string)  [unwired: 4 in, 2 out]
      n684 = call "Extract String.vi"("Resolution"=w1731, "Condition"=w1734) -> ("배열 1"=w1730:string[], "배열 2"=w1748:string[])  [unwired: 7 in, 1 out]
      n685 = Index Array(array=w1730) -> (element #2=w1728:string)  [unwired: 2 in, 1 out]
      n686 = Insert Into Array(array=w1748, new element=w1728) -> (w1729:string[])  [unwired: 1 in]
      n687 = call-poly "String Contents.vi"("문자 배열"=w1729, "참조 배열"=w1752, "에러 입력"=w1732) -> ("에러 출력"=w1727:errorcluster)  [unwired: 7 in, 1 out]
      n688 = call "Certi Recall.vi"("큐 입력"=w1760, "NumRows"=w1754, "입력 클러스터"=w1753, "에러 입력"=w1727, "Func_ext in"=w1740) -> ("에러 출력"=w1755:errorcluster)  [unwired: 5 in, 1 out]
    }
    frame "Flatness_1" {
      n689 = call "Get Calproc.vi"("제목"=w1822, "에러 입력"=w1820, "Func_ext"=w1821) -> ("에러 출력"=w1841:errorcluster, "Condition"=w1794:string[][], "Func_ext Out"=w1840:string, "클러스터"=w1836:T7)  [unwired: 5 in]
      n690 = Unbundle By Name(w1823) -> ("Initialize 1.Spec"=w1811:refnum<vi>[], "Initialize 2.문자열"=w1788:refnum<vi>[], "Initialize 2.콤보박스"=w1805:refnum<vi>[], "Initialize 1.Condition"=w1810:refnum<vi>[])
      n691 = Unbundle By Name(w1836) -> ("Data"=w1799:string[][], "Spec"=w1837:string[][], "CMC"=w1832:string[][], "NumRows"=w1818:u32)
      n692 = call "Variables Data IO.vi"("Select"=Cmd_Var_Data_IO."Condition Default", "error in"=w1841, "Data In"=w1794, "Func_ext"=w1840) -> ("error out"=w1835:errorcluster, "Func_ext Out"=w1829:string)  [unwired: 5 in, 1 out]
      n693 = Index Array(array=w1799, index (col)=7 ("비활성화된 인덱스 (열)")) -> (element=w1797:string[])  [unwired: 1 in]
      n694 = Insert Into Array(array=w1794, index (col)=0 ("비활성화된 인덱스 (열)"), new element=w1797) -> (w1795:string[][])  [unwired: 1 in]
      n695 = Index Array(array=w1810) -> (element=w1833:refnum<vi>)  [unwired: 1 in]
      n696 = call "Variables Data IO.vi"("Select"=Cmd_Var_Data_IO."Condition", "error in"=w1835, "Data In"=w1795, "Func_ext"=w1829) -> ("error out"=w1813:errorcluster, "Func_ext Out"=w1809:string)  [unwired: 5 in, 1 out]
      n697 = Index Array(array=w1805) -> (element=w1814:refnum<vi>)  [unwired: 1 in]
      n698 = call-poly "Table Initialize.vi"("행의 개수"=w1818, "Table Ref"=w1833, "Value"=w1795, "에러 입력"=w1813) -> ("에러 출력"=w1812:errorcluster)  [unwired: 5 in, 2 out]
      n699 = call "Select E_M Range.vi"("STD Select Ref."=w1814, "에러 입력"=w1812, "Func in"=w1809) -> ("에러 출력"=w1816:errorcluster, "STD Select Value"=w1815:string, "Func out"=w1808:string)  [unwired: 5 in, 1 out]
      n700 = call "STD Cal Data.vi"("error in"=w1816, "문자열"=w1815, "Func_ext"=w1808) -> ("error out"=w1791:errorcluster, "Data Out"=w1804:string[][], "Func_ext Out"=w1807:string)  [unwired: 4 in, 2 out]
      n701 = Index Array(array=w1804, index (row)=0 ("인덱스 (행)"), index (col)=24 ("비활성화된 인덱스 (열)")) -> (element=w1793:string)
      n702 = Build Array(w1793) -> (w1792:string[])
      n703 = call-poly "String Contents.vi"("문자 배열"=w1792, "참조 배열"=w1788, "에러 입력"=w1791) -> ("에러 출력"=w1790:errorcluster)  [unwired: 7 in, 1 out]
      n704 = for {
        tunnel: w1794 -> [w1847] mode=indexing
        tunnel: [w1846] -> w1801 mode=indexing
        tunnel: w1793 -> [w1851]
        tunnel: [w1848] -> w1800 mode=indexing
        tunnel: w1799 -> [w1845] mode=indexing
        n705 = Index Array(array=w1845, index #1=5 ("인덱스")) -> (element #1=w1843:string, element #2=w1842:string)  [unwired: 1 in]
        n706 = Build Array("Digital" ("원소"), w1851, "μm" ("원소")) -> (w1848:string[])
        n707 = Build Array (concatenate)(w1847, w1843, w1842) -> (w1846:string[])
      }
      n708 = Index Array(array=w1811) -> (element=w1834:refnum<vi>)  [unwired: 1 in]
      n709 = call "Create Resolution.vi"("행의 개수"=w1818, "에러 입력(에러 없음)"=w1790, "Resolution"=w1800, "Func_ext"=w1807) -> ("에러 출력"=w1828:errorcluster, "Resolution Out"=w1838:string[][], "Func_ext 출력"=w1839:string)  [unwired: 5 in]
      n710 = call "Get Spec.vi"("NumRows"=w1818, "Spec in"=w1837, "Spec Ref."=w1834, "error in"=w1828, "Condition in"=w1801, "Resolution in"=w1838, "Func_ext"=w1839) -> ("error out"=w1827:errorcluster, "Data Out"=w1831:string[][], "Func_ext Out"=w1830:string)  [unwired: 2 out]
      n711 = call "Match_CMC.vi"("CMC IN"=w1832, "error in"=w1827, "Condition IN"=w1831, "Func_ext"=w1830) -> ("error out"=w1789:errorcluster, "Func_ext out"=w1806:string)  [unwired: 4 in, 2 out]
      n712 = call "Certi Recall.vi"("큐 입력"=w1824, "NumRows"=w1818, "입력 클러스터"=w1817, "에러 입력"=w1789, "Func_ext in"=w1806) -> ("에러 출력"=w1819:errorcluster)  [unwired: 5 in, 1 out]
    }
    frame "Straightness_1" {
      n713 = Unbundle By Name(w1884) -> ("Initialize 2.콤보박스"=w1864:refnum<vi>[], "Initialize 2.문자열"=w1875:refnum<vi>[], "Initialize 1.Condition"=w1876:refnum<vi>[], "Initialize 1.Spec"=w1894:refnum<vi>[], "Initialize 1.Resolution"=w1893:refnum<vi>[], "Initialize 1.Measured"=w1855:refnum<vi>[])
      n714 = call "Get Calproc.vi"("제목"=w1883, "에러 입력"=w1881, "Func_ext"=w1882) -> ("에러 출력"=w1904:errorcluster, "Condition"=w1902:string[][], "Func_ext Out"=w1903:string, "클러스터"=w1898:T7)  [unwired: 5 in]
      n715 = Unbundle By Name(w1898) -> ("Resolution"=w1896:string[][], "Spec"=w1899:string[][], "CMC"=w1895:string[][], "Data"=w1853:string[][], "NumRows"=w1879:u32, "Condition"=w1869:string[][], "Resolution"=w1867:string[][])
      n716 = call "Extract String.vi"("Resolution"=w1867, "Condition"=w1869) -> ("배열 1"=w1870:string[], "배열 2"=w1868:string[])  [unwired: 7 in, 1 out]
      n717 = Index Array(array=w1893) -> (element=w1857:refnum<vi>)  [unwired: 1 in]
      n718 = call "Variables Data IO.vi"("Select"=Cmd_Var_Data_IO."Condition", "error in"=w1904, "Data In"=w1853, "Func_ext"=w1903) -> ("error out"=w1897:errorcluster, "Func_ext Out"=w1890:string)  [unwired: 5 in, 1 out]
      n719 = Index Array(array=w1894) -> (element=w1856:refnum<vi>)  [unwired: 1 in]
      n720 = call "Variables Data IO.vi"("Select"=Cmd_Var_Data_IO."Condition Default", "error in"=w1897, "Data In"=w1902, "Func_ext"=w1890) -> ("error out"=w1905:errorcluster, "Func_ext Out"=w1906:string)  [unwired: 5 in, 1 out]
      n721 = Index Array(array=w1876) -> (element #1=w1858:refnum<vi>)  [unwired: 2 in, 1 out]
      n722 = call "Create Resolution.vi"("행의 개수"=w1879, "Table Ref"=w1857, "에러 입력(에러 없음)"=w1905, "Resolution"=w1896, "Func_ext"=w1906) -> ("에러 출력"=w1889:errorcluster, "Resolution Out"=w1900:string[][], "Func_ext 출력"=w1901:string)  [unwired: 4 in]
      n723 = call "Get Spec.vi"("NumRows"=w1879, "Spec in"=w1899, "Spec Ref."=w1856, "error in"=w1889, "Condition in"=w1902, "Resolution in"=w1900, "Func_ext"=w1901) -> ("error out"=w1888:errorcluster, "Data Out"=w1892:string[][], "Func_ext Out"=w1891:string)  [unwired: 2 out]
      n724 = call "Match_CMC.vi"("CMC IN"=w1895, "error in"=w1888, "Condition IN"=w1892, "Func_ext"=w1891) -> ("error out"=w1863:errorcluster, "Func_ext out"=w1874:string)  [unwired: 4 in, 2 out]
      n725 = call "STD Cal Data.vi"("error in"=w1863, "Func_ext"=w1874) -> ("error out"=w1862:errorcluster, "Func_ext Out"=w1877:string)  [unwired: 5 in, 3 out]
      n726 = call "Array Size.vi"("Data in"=w1853) -> ("열(U32)"=w1861:u32)  [unwired: 7 in, 3 out]
      n727 = call-poly "Table Initialize.vi"("행의 개수"=w1879, "Table Ref"=w1858, "Value"=w1853, "에러 입력"=w1862, "열의 개수"=w1861) -> ("에러 출력"=w1852:errorcluster)  [unwired: 4 in, 2 out]
      n728 = Build Array (concatenate)(w1858, w1857, w1856, w1855) -> (w1854:refnum<vi>[])
      n729 = call "Tbl Comp.vi"("배열"=w1854, "방향"=enum16{"수직", "수평"}."수평", "에러 입력"=w1852) -> ("에러 출력"=w1860:errorcluster)  [unwired: 6 in, 2 out]
      n730 = call-poly "String Contents.vi"("문자 배열"=w1868, "참조 배열"=w1875, "에러 입력"=w1860) -> ("에러 출력"=w1866:errorcluster)  [unwired: 7 in, 1 out]
      n731 = call-poly "String Contents.vi"("문자 배열"=w1870, "참조 배열"=w1864, "에러 입력"=w1866) -> ("에러 출력"=w1872:errorcluster, "참조"=w1871:refnum<vi>)  [unwired: 7 in]
      n732 = property on="표시형식" class="CmbBox"(reference=w1871, error in=w1872, "Strings[]"=w1873) -> (error out=w1865:errorcluster)  [unwired: 1 out]
      n733 = call "Certi Recall.vi"("큐 입력"=w1885, "NumRows"=w1879, "입력 클러스터"=w1878, "에러 입력"=w1865, "Func_ext in"=w1877) -> ("에러 출력"=w1880:errorcluster)  [unwired: 5 in, 1 out]
    }
    frame Default {
    }
  }
  "error out" <- w6
  "data 1 (2d)" <- w16
  "data 2 (3d)" <- w1
  n734 = Unbundle By Name(w6) -> ("status"=w14:bool)
  n735 = Not(x=w14) -> (.not. x?=→"Load?":bool)
